vi "Viavi - Main.vi"(8 "error in (no error)":errorcluster {"code" format="Error %.0f"}, 10 "notifiers":T8, 11 "messageQueues":T9) -> (0 "error out":errorcluster {"code" format="Error %.0f"})   [LabVIEW 2017]
uses:
  Support/Configuration/Message Queues/messageQueues.ctl
  Support/Configuration/Message Queues/Message Cluster.ctl
  Support/Configuration/Notifiers/notifiers.ctl
  Controls/Viavi - Data.ctl
  Controls/Viavi - objectRefs.ctl
  Controls/Viavi - Instructions.ctl
  75e8a571-c33f-46d4-930b-ea0aecc2dba4.vi
  c46a4b58-3cb9-4cd0-a122-5f2cefd5d860.vi
  <vilib>/Utility/error.llb/Error Cluster From Error Code.vi
  <vilib>/ErrorRing/Error Ring.xnode
  Support/Configuration/User Events/User Event - Stop.lvlib
  Support/Configuration/Message Queues/Message Queue.lvlib
  <instrlib>/Viavi mORL-A1/Viavi mORL-A1.lvlib
  Support/Configuration/Notifiers/notifiers.lvlib
panel:
  in  "IL Warnings Enable":bool
  in  "IL Warning Values":cluster{"IL Min":dbl, "IL Max":dbl}={"IL Min"=0.0, "IL Max"=99.0}
  in  "Table Key":cluster{"Warning":bool, "Failure":bool}
  out "Data Error":string
  out "Method Selection":u16(ring) items=["Select Test Method", "---------------------", "Standard", "Substitution", "Cutback (placeholder)"]
  out "Testing Parameters":T1={"IL Param"={"Warning High"=inf, "Warning Low"=0.0, "Fail High"=0.0, "Fail Low"=-inf, "Display Precision"=2}, "RL Param"={"Warning High"=inf, "Warning Low"=35.0, "Fail High"=inf, "Fail Low"=0.0, "Display Precision"=1}, "RL2 Param"={"Warning High"=inf, "Warning Low"=35.0, "Fail High"=inf, "Fail Low"=-inf, "Display Precision"=1}, "Power Param"={"Warning High"=inf, "Warning Low"=-28.0, "Fail High"=inf, "Fail Low"=-inf, "Display Precision"=2}, "Length Param"={"Warning High"=inf, "Warning Low"=-inf, "Fail High"=inf, "Fail Low"=-inf, "Display Precision"=1}}
  out "pRatio Array":dbl[](array[numeric])
  out "Temp Ref Power Array":T2(array[cluster])
  out "Temp Power Array":T2(array[cluster])
  out "Temp RL2 Array":T2(array[cluster])
  out "Temp RL Array":T2(array[cluster])
  out "Temp IL Array":T2(array[cluster])
  out "Length Array":T2(array[cluster])
  out "Ref Length Array":T2(array[cluster])
  in  "Measure pRatio":bool
  in  "First Reference":bool=TRUE caption="Taken First Ref"
  out "Single Channel":bool
  out "Enable RL":bool
  out "Enable IL":bool
  out "Wavelength Enable":bool[](array[boolean])
  out "Channel Select":bool[](array[boolean])
  out "Has Switch":bool caption="Switch Installed"
  in  "Slot Number":i32=3
  out "Device ID":refnum<visa-resource-name>="GPIB0::17::INSTR"
  in  "displayTab":T3(tab)
  in  "Custom RL Cluster":T4 {"RL Method" items=["", "Input", "Output", "Between", "In + Out"]}
  in  "RL2 Standard":u16(ring) items=["Select RL2 Standard", "---------------------", "No Standard", "Custom Standard", "---------------------", "GR326-UPC-New ", "GR326-UPC-During/End", "GR326-APC-New ", "GR326-APC-During/End", "GR1435-Standard-New", "GR1435-Standard-During/End"]
  out "Both Image":picture
  out "Between Image":picture
  out "Output Image":picture
  out "Input Image":picture
  out "RL Presets":T5(radio)
  out "RL Configs":T6={"Measurement Mode"=FALSE, "Enable RL2"=FALSE, "RL1 Anchor Point"=enum."Left DUT Connection", "RL1 Measure Points"={-0.2500000000000009, 0.25}, "RL2 Anchor Point"=enum."Right DUT Connection", "RL2 Measure Points"={-0.2500000000000009, 0.25}} {"RL2 Measure Points" scale=-5.0..5.0 scale format="%#.2g"; "RL1 Measure Points" scale=-5.0..5.0 scale format="%#.2g"}
  out "Single Table":T7(array[cluster])
  out "Multi Ref/IL Table":T7(array[cluster])
  out "Multi RL Table":T7(array[cluster])
  out "Multi Ref/IL Columns":T2(array[cluster])=[{"String"="", "Warning"=FALSE, "Fail"=FALSE, "Numeric"=0.0}, {"String"="Ref: 1310", "Warning"=FALSE, "Fail"=FALSE, "Numeric"=0.0}, {"String"="Ref: 1490", "Warning"=FALSE, "Fail"=FALSE, "Numeric"=0.0}, {"String"="Ref: 1550", "Warning"=FALSE, "Fail"=FALSE, "Numeric"=0.0}, {"String"="Ref: 1625", "Warning"=FALSE, "Fail"=FALSE, "Numeric"=0.0}, {"String"="IL: 1310", "Warning"=FALSE, "Fail"=FALSE, "Numeric"=0.0}, {"String"="IL: 1490", "Warning"=FALSE, "Fail"=FALSE, "Numeric"=0.0}, {"String"="IL: 1550", "Warning"=FALSE, "Fail"=FALSE, "Numeric"=0.0}, {"String"="IL: 1625", "Warning"=FALSE, "Fail"=FALSE, "Numeric"=0.0}]
  out "Multi RL Columns":T2(array[cluster])=[{"String"="", "Warning"=FALSE, "Fail"=FALSE, "Numeric"=0.0}, {"String"="RL: 1310", "Warning"=FALSE, "Fail"=FALSE, "Numeric"=0.0}, {"String"="RL: 1490", "Warning"=FALSE, "Fail"=FALSE, "Numeric"=0.0}, {"String"="RL: 1550", "Warning"=FALSE, "Fail"=FALSE, "Numeric"=0.0}, {"String"="RL: 1625", "Warning"=FALSE, "Fail"=FALSE, "Numeric"=0.0}, {"String"="RL2: 1310", "Warning"=FALSE, "Fail"=FALSE, "Numeric"=0.0}, {"String"="RL2: 1490", "Warning"=FALSE, "Fail"=FALSE, "Numeric"=0.0}, {"String"="RL2: 1550", "Warning"=FALSE, "Fail"=FALSE, "Numeric"=0.0}, {"String"="RL2: 1625", "Warning"=FALSE, "Fail"=FALSE, "Numeric"=0.0}]
  in  "Instruction Button":bool
  out "Instruction Image":picture
  out "Instruction Text":string
  # "Custom RL\nOption"
  # "Select which point to measure"
  # "(if applicable)"
  # "Discrete"
  # "Integral"
  # "Left Point"
  # "Right Point"
  # "Left Point"
  # "Right Point"
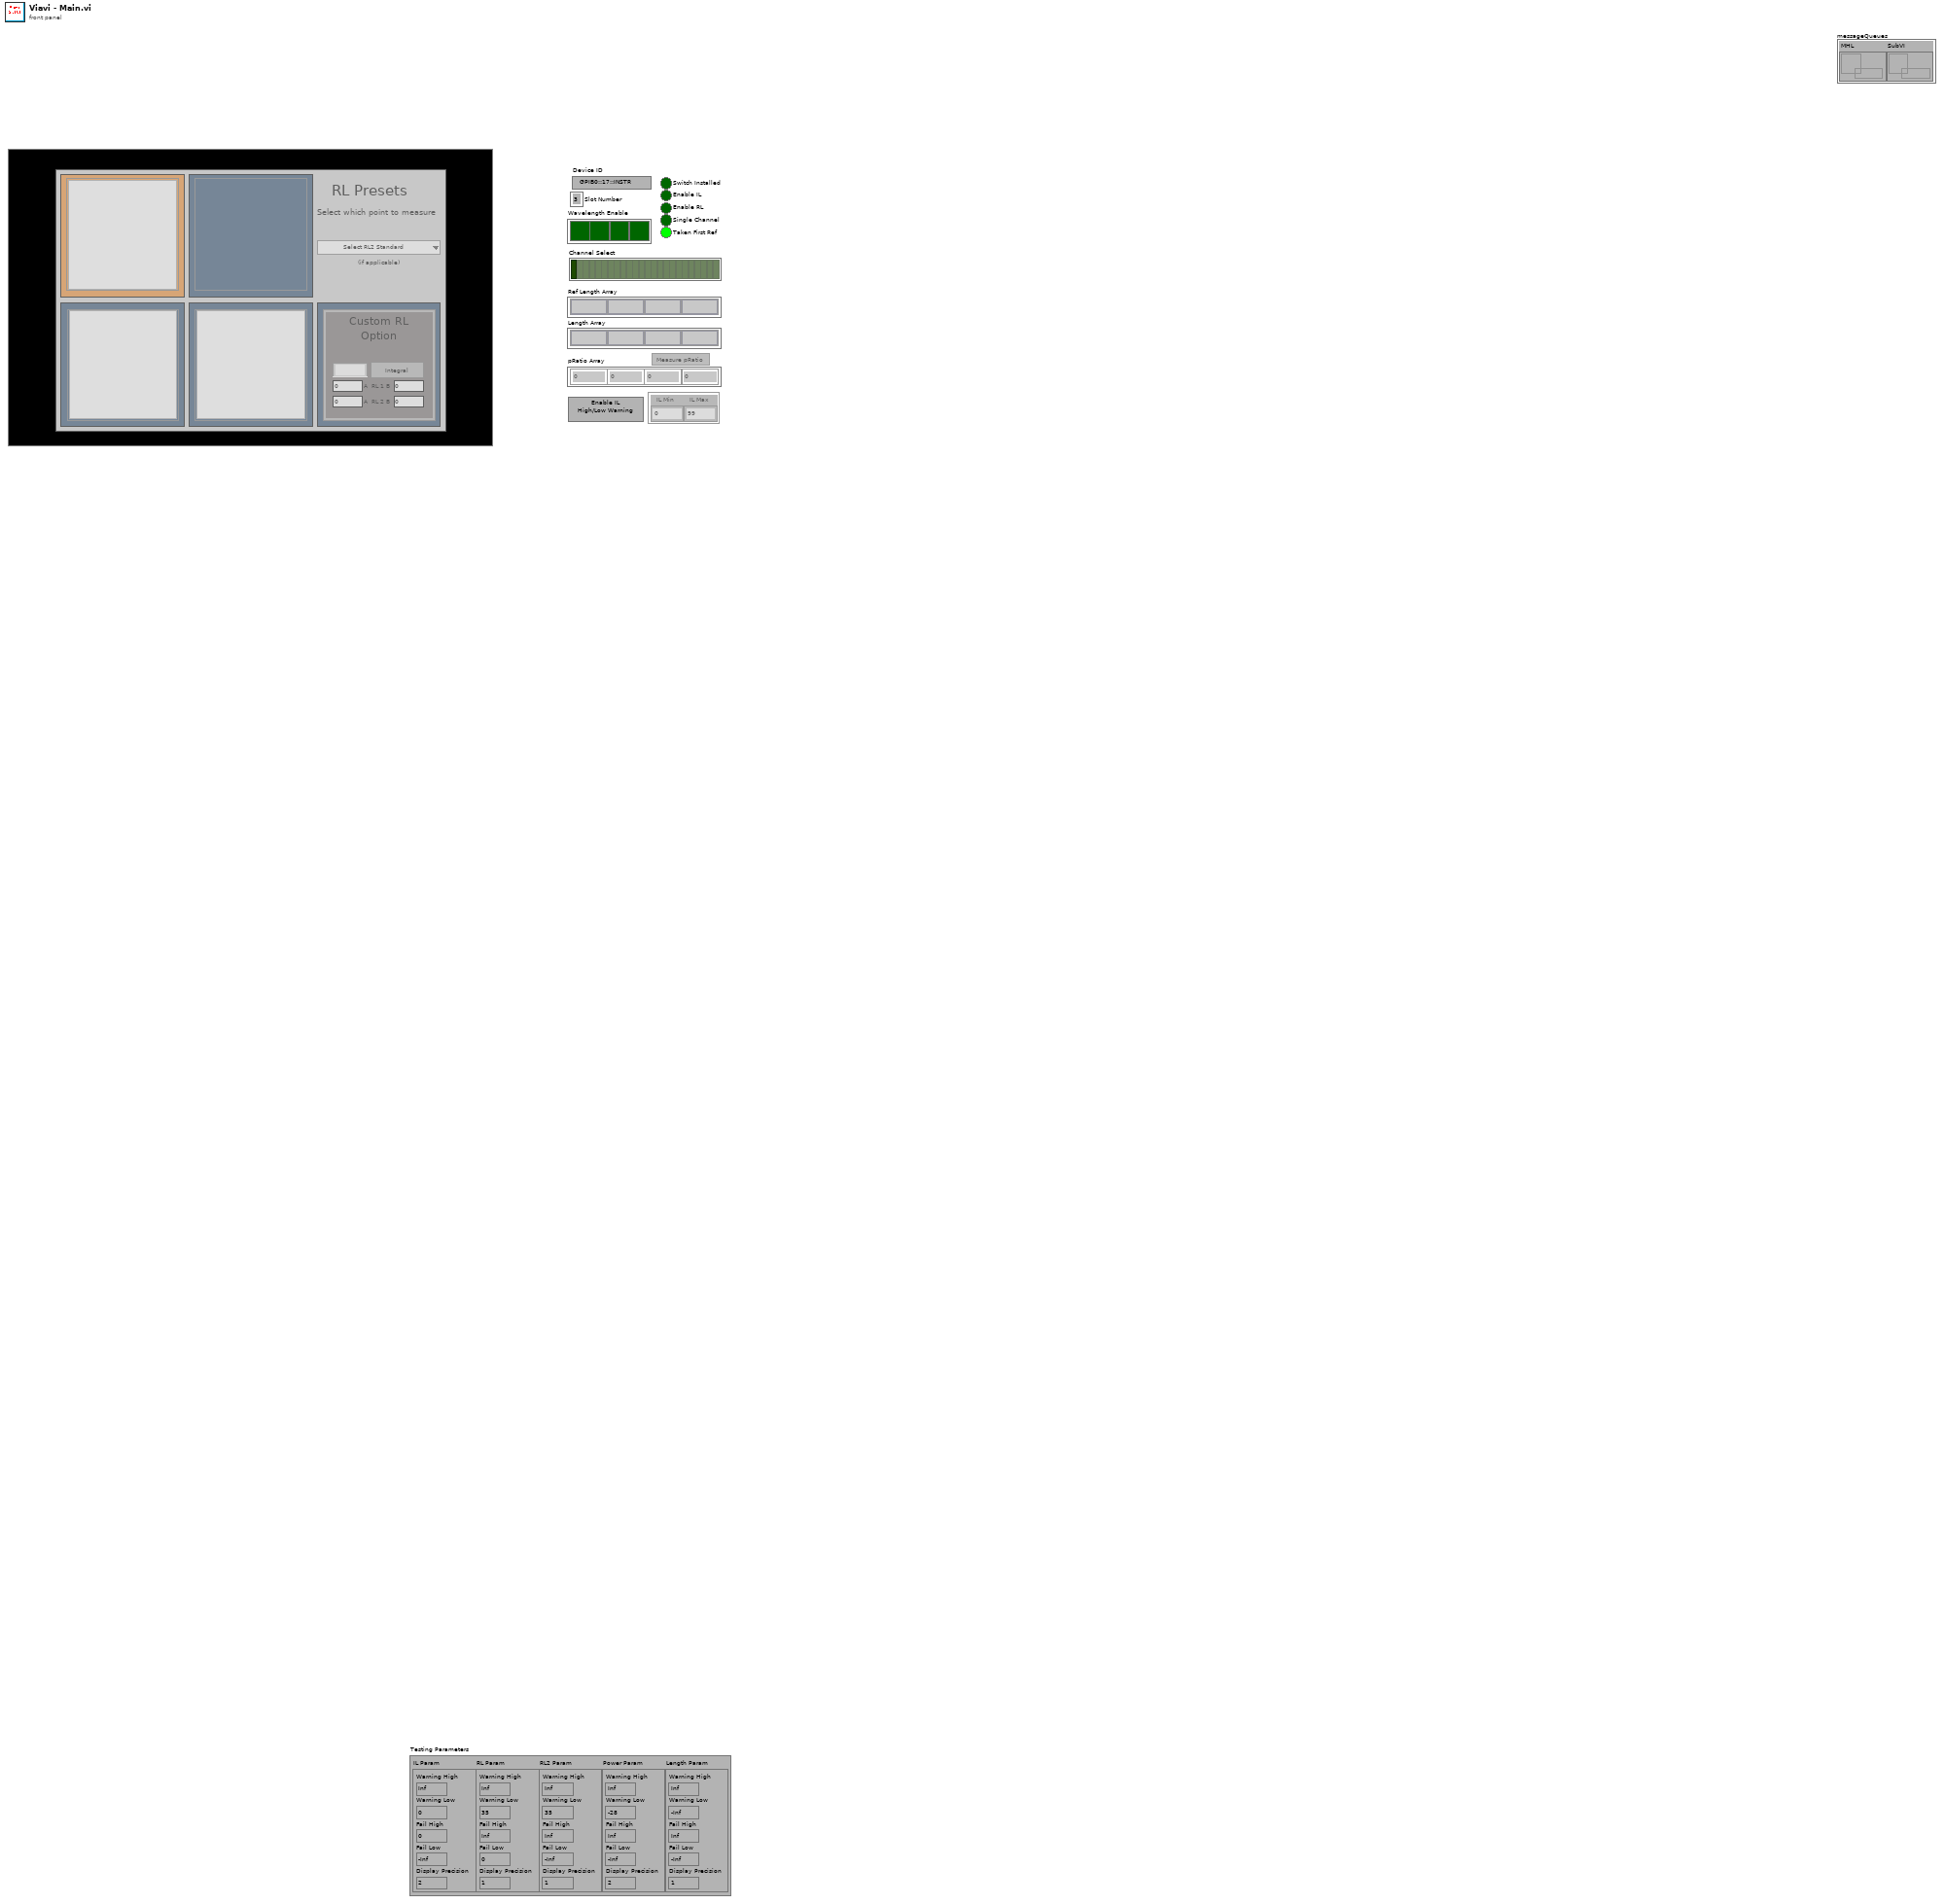
[diagram p1: front panel]
types:
  T1 = cluster{"IL Param":cluster{"Warning High":dbl, "Warning Low":dbl, "Fail High":dbl, "Fail Low":dbl, "Display Precision":i32}, "RL Param":cluster{"Warning High":dbl, "Warning Low":dbl, "Fail High":dbl, "Fail Low":dbl, "Display Precision":i32}, "RL2 Param":cluster{"Warning High":dbl, "Warning Low":dbl, "Fail High":dbl, "Fail Low":dbl, "Display Precision":i32}, "Power Param":cluster{"Warning High":dbl, "Warning Low":dbl, "Fail High":dbl, "Fail Low":dbl, "Display Precision":i32}, "Length Param":cluster{"Warning High":dbl, "Warning Low":dbl, "Fail High":dbl, "Fail Low":dbl, "Display Precision":i32}}
  T2 = cluster{"String":string, "Warning":bool, "Fail":bool, "Numeric":dbl}[]
  T3 = enum32{"RL Configs", "Data Table", "Instruction"}
  T4 = cluster{"Enable Integral":bool, "RL 1 A":dbl, "RL 1 B":dbl, "RL 2 A":dbl, "RL 2 B":dbl, "Enable RL2":bool, "RL Method":u16}
  T5 = enum32{"Left Anchor", "Right Anchor", "Center Anchor", "Left/Right Anchor", "Custom"}
  T6 = cluster{"Measurement Mode":bool, "Enable RL2":bool, "RL1 Anchor Point":enum32{"Left DUT Connection", "Right DUT Connection", "Center on DUT"}, "RL1 Measure Points":cluster{dbl, dbl}, "RL2 Anchor Point":enum32{"Left DUT Connection", "Right DUT Connection", "Center on DUT"}, "RL2 Measure Points":cluster{dbl, dbl}}
  T7 = cluster{"String":string, "Warning":bool, "Fail":bool, "Numeric":dbl}[][]
  T8 = typedef "notifiers.lvlib/notifiers.ctl" = cluster{"exitSubVI":refnum<notifier>}
  T9 = typedef "Message Queue.lvlib/messageQueues.ctl" = cluster{"MHL":refnum<queue>, "SubVI":refnum<queue>}
  T10 = typedef "Viavi - Data.ctl" = cluster{"Viavi - objectRefs":T11}
  T11 = typedef "Viavi - objectRefs.ctl" = cluster{"displayTab":refnum<vi>, "SubVI Pane":refnum<vi>, "instructStringRef":refnum<vi>, "instructImageRef":refnum<vi>, "instructButtonRef":refnum<vi>, "ResourceNameRef":refnum<vi>, "SlotNumberRef":refnum<vi>, "HasSwitchRef":refnum<vi>, "WavelengthRef":refnum<vi>, "SingleChannelRef":refnum<vi>, "IlEnableRef":refnum<vi>, "RlEnableRef":refnum<vi>, "RLConfigsRef":refnum<vi>, "RLPresetRef":refnum<vi>, "SingleTableRef":refnum<vi>, "MultiRef/ILTableRef":refnum<vi>, "MultiRLTableRef":refnum<vi>, "TempILRef":refnum<vi>, "TempRLRef":refnum<vi>, "TempRL2Ref":refnum<vi>, "TempRefPowRef":refnum<vi>, "TempPowRef":refnum<vi>, "RefLengthRef":refnum<vi>, "LengthArrayRef":refnum<vi>, "ChannelRef":refnum<vi>, "TestParamsRef":refnum<vi>, "MethodSelectRef":refnum<vi>, "DataErrorRef":refnum<vi>, "RL2StandardRef":refnum<vi>}
  T12 = typedef "User Event - Stop.lvlib/userEvents.ctl" = cluster{"stop":refnum<user-event>, "sendRefs":refnum<user-event>, "sendSubVIRefs":refnum<user-event>, "eventRegRef":refnum<event-registration>}
  T13 = cluster{"queueName":string, "queueMessage":string, "priority?":bool}[]
  T14 = enum8{"Enabled", "Disabled", "Disabled and Grayed Out"}
  T15 = cluster{"VISA resource name":refnum<visa-resource-name>, "HasSwitch":bool}
  T16 = cluster{"Wavelength Enable":bool[], "Channel Cluster":bool[], "Enable IL":bool, "Enable RL":bool, "Enable Switch":bool, "Method Selection":u16, "Value":cluster{"Standard Name":string, "Max IL to Pass (dB)":dbl, "Min RL to Pass (dB)":dbl}}
  T17 = typedef "Viavi - Instructions.ctl" = cluster{"Reference Instructions":cluster{"Instruction Text":string, "Instruction Image":picture, "Main Display Message":string}, "Reference (substitution) Instructions":cluster{"Instruction Text":string, "Instruction Image":picture, "Main Display Message":string}, "Reference (cutback) Instructions":cluster{"Instruction Text":string, "Instruction Image":picture, "Main Display Message":string}, "Measure Instructions":cluster{"Instruction Text":string, "Instruction Image":picture, "Main Display Message":string}, "Measure (Substitution) Instructions":cluster{"Instruction Text":string, "Instruction Image":picture, "Main Display Message":string}, "Measure (Cutback) Instructions":cluster{"Instruction Text":string, "Instruction Image":picture, "Main Display Message":string}, "Disconnect Int Sphere Instructions":cluster{"Instruction Text":string, "Instruction Image":picture, "Main Display Message":string}, "Connect Int Sphere Instructions":cluster{"Instruction Text":string, "Instruction Image 2":picture, "Main Display Message":string}, " Multichannel Reference Instructions":cluster{"Instruction Text":string, "Instruction Image":picture, "Main Display Message":string}, " Multichannel Reference (substitution) Instructions":cluster{"Instruction Text":string, "Instruction Image":picture, "Main Display Message":string}, " Multichannel Reference (cutback) Instructions":cluster{"Instruction Text":string, "Instruction Image":picture, "Main Display Message":string}, "Multichannel Measure Instructions":cluster{"Instruction Text":string, "Instruction Image":picture, "Main Display Message":string}, "Multichannel Measure (Substitution) Instructions":cluster{"Instruction Text":string, "Instruction Image":picture, "Main Display Message":string}, "Multichannel Measure (Cutback) Instructions":cluster{"Instruction Text":string, "Instruction Image":picture, "Main Display Message":string}}
  T18 = cluster{"Temp Ref Power Array":cluster{"String":string, "Warning":bool, "Fail":bool, "Numeric":dbl}[], "Temp IL Array":cluster{"String":string, "Warning":bool, "Fail":bool, "Numeric":dbl}[], "Temp RL Array":cluster{"String":string, "Warning":bool, "Fail":bool, "Numeric":dbl}[], "Temp RL2 Array":cluster{"String":string, "Warning":bool, "Fail":bool, "Numeric":dbl}[]}
  T19 = cluster{"IL Array":cluster{"Data Output":string, "Fail":bool}[], "RL Array":cluster{"Data Output":string, "Fail":bool}[], "Ref Power Array":string[], "Power Array":string[], "Optional Data Array":cluster{"Data Output":string, "Fail":bool}[], "Optional Param":string}
  T20 = cluster{"Standard Name":string, "Max IL to Pass (dB)":dbl, "Min RL to Pass (dB)":dbl}
  T21 = cluster{"String":string, "Warning":bool, "Fail":bool, "Numeric":dbl}
  T22 = cluster{"Measurement Mode":bool, "Enable RL2":bool, "RL1 Anchor Point":enum32{"Left DUT Connection", "Right DUT Connection", "Center on DUT"}, "RL1 Measure Points":cluster{"RL1 Left":dbl, "RL1 Right":dbl}, "RL2 Anchor Point":enum32{"Left DUT Connection", "Right DUT Connection", "Center on DUT"}, "RL2 Measure Points":cluster{"RL2 Left":dbl, "RL2 Right":dbl}}
  T23 = cluster{"Instruction Text":string, "Instruction Image":picture, "Main Display Message":string}[]
  T24 = cluster{"Instruction Text":string, "Instruction Image":picture, "Main Display Message":string}
  T25 = cluster{"Temp IL Array":cluster{"String":string, "Warning":bool, "Fail":bool, "Numeric":dbl}[], "Temp RL Array":cluster{"String":string, "Warning":bool, "Fail":bool, "Numeric":dbl}[], "Temp RL2 Array":cluster{"String":string, "Warning":bool, "Fail":bool, "Numeric":dbl}[], "Temp Power Array":cluster{"String":string, "Warning":bool, "Fail":bool, "Numeric":dbl}[], "Length Array":cluster{"String":string, "Warning":bool, "Fail":bool, "Numeric":dbl}[]}
  T26 = cluster{"Warning High":dbl, "Warning Low":dbl, "Fail High":dbl, "Fail Low":dbl, "Display Precision":i32}
  T27 = cluster{"Standard Name":string, "Max IL to Pass (dB)":dbl, "Min RL to Pass (dB)":dbl}[]
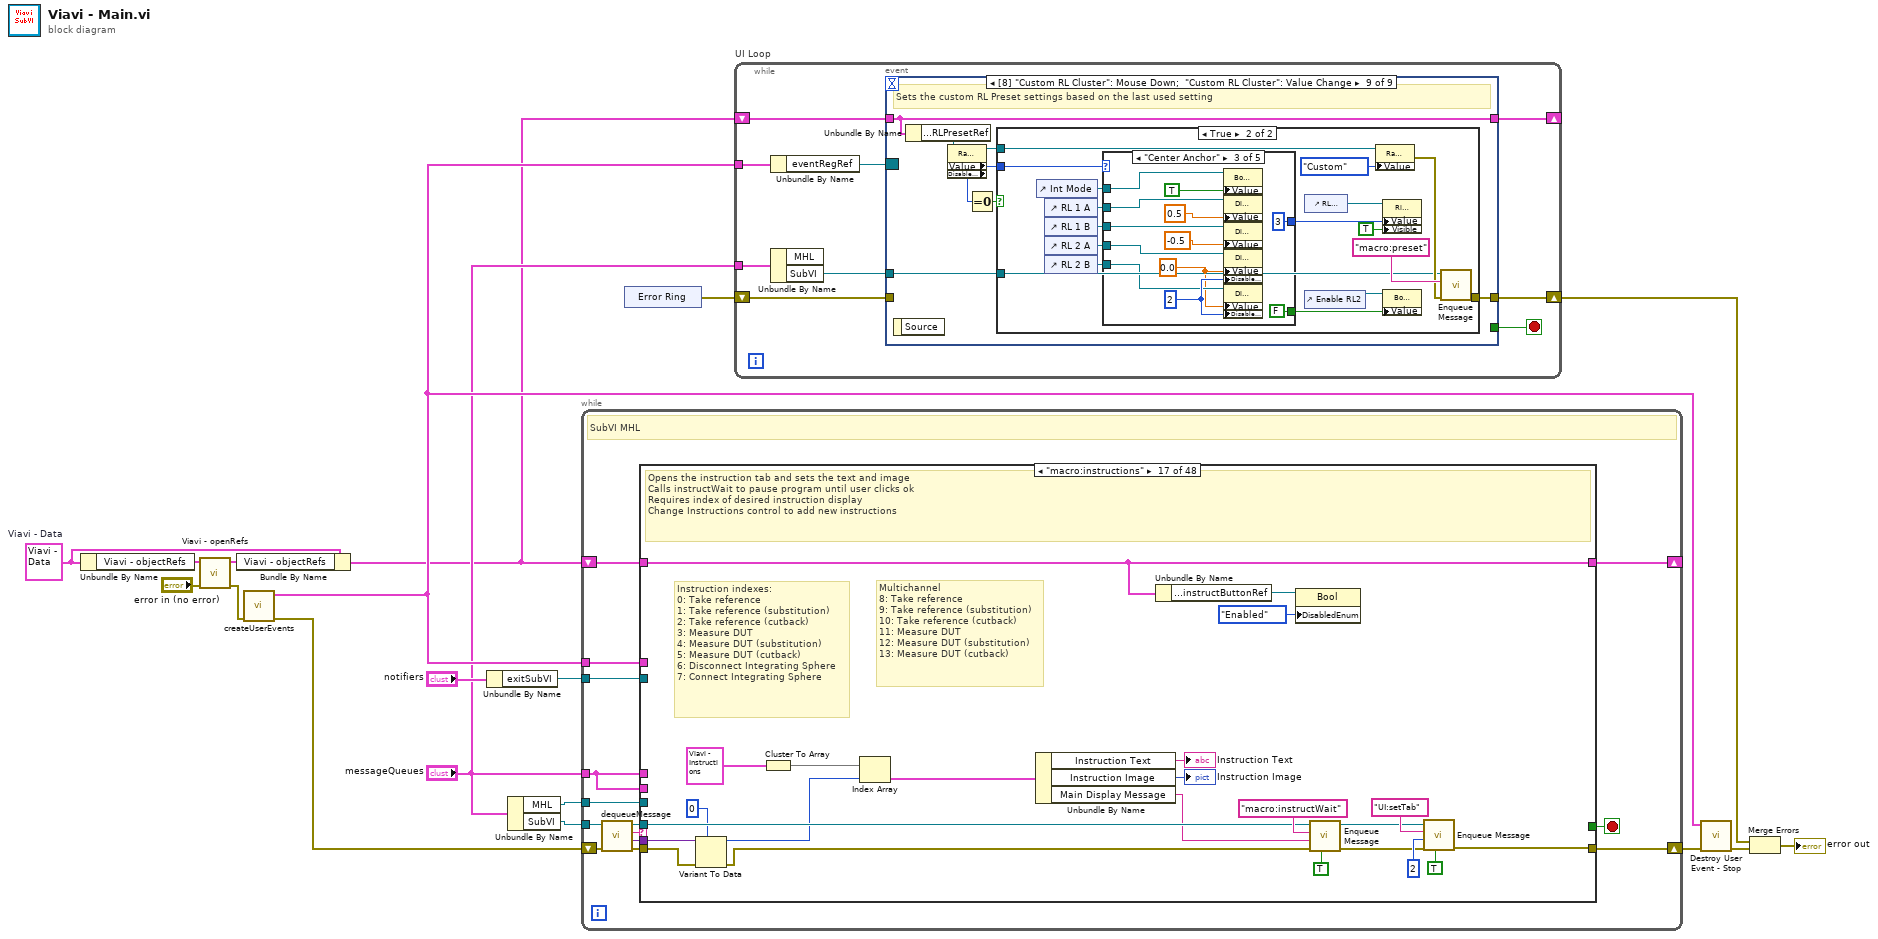
[diagram p0: block diagram]
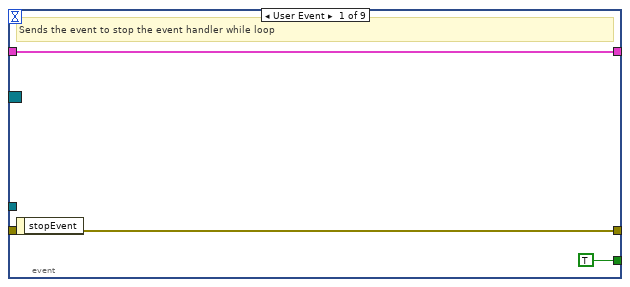
[diagram p2: hidden frame]
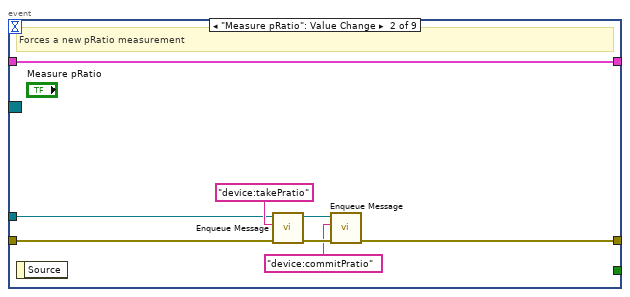
[diagram p3: hidden frame]
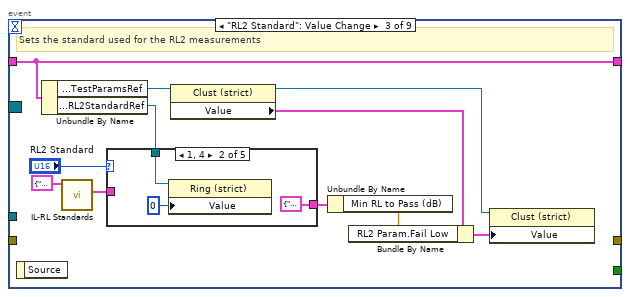
[diagram p4: hidden frame]
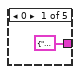
[diagram p5: hidden frame]
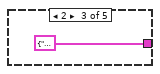
[diagram p6: hidden frame]
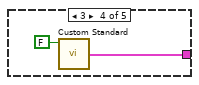
[diagram p7: hidden frame]
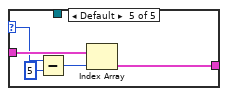
[diagram p8: hidden frame]
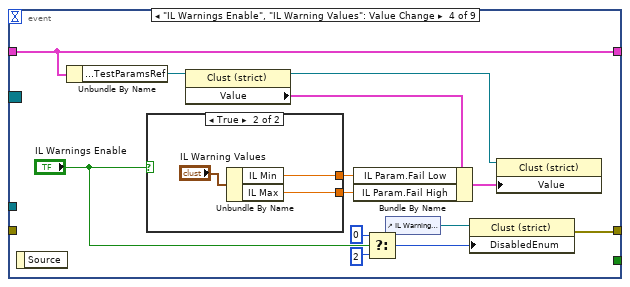
[diagram p9: hidden frame]
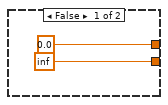
[diagram p10: hidden frame]
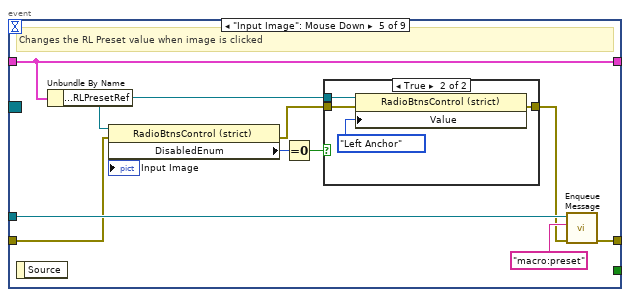
[diagram p11: hidden frame]
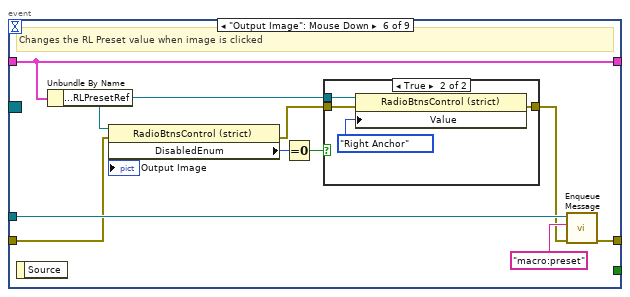
[diagram p13: hidden frame]
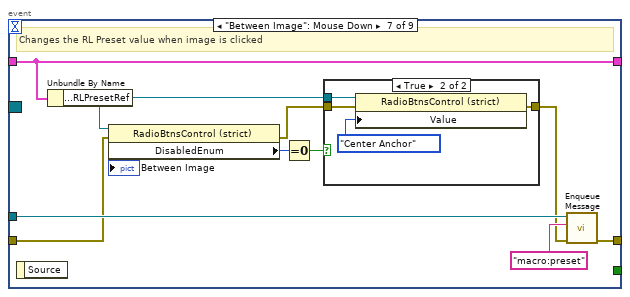
[diagram p15: hidden frame]
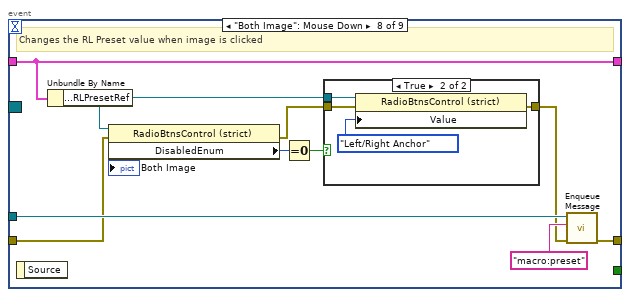
[diagram p17: hidden frame]
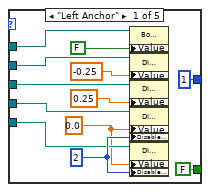
[diagram p20: hidden frame]
diagram:
  w5 = T10 {"Viavi - objectRefs"={"displayTab"=refnum, "SubVI Pane"=refnum, "instructStringRef"=refnum, "instructImageRef"=refnum, "instructButtonRef"=refnum, "ResourceNameRef"=refnum, "SlotNumberRef"=refnum, "HasSwitchRef"=refnum, "WavelengthRef"=refnum, "SingleChannelRef"=refnum, "IlEnableRef"=refnum, "RlEnableRef"=refnum, "RLConfigsRef"=refnum, "RLPresetRef"=refnum, "SingleTableRef"=refnum, "MultiRef/ILTableRef"=refnum, "MultiRLTableRef"=refnum, "TempILRef"=refnum, "TempRLRef"=refnum, "TempRL2Ref"=refnum, "TempRefPowRef"=refnum, "TempPowRef"=refnum, "RefLengthRef"=refnum, "LengthArrayRef"=refnum, "ChannelRef"=refnum, "TestParamsRef"=refnum, "MethodSelectRef"=refnum, "DataErrorRef"=refnum, "RL2StandardRef"=refnum}}  # Viavi - Data
  n1 = Unbundle By Name(w5) -> ("Viavi - objectRefs"=w6:T11)
  n2 = call "Viavi - openRefs.vi"("error in (no error)"="error in (no error)", "Viavi - strictRefs In"=w6) -> ("error out"=w2:errorcluster, "Viavi - strictRefs Out"=w4:T11)  [unwired: 6 in, 2 out]
  n3 = Bundle By Name(cluster=w5, "Viavi - objectRefs"=w4) -> (w1:T10)
  n4 = call "createUserEvents.vi"("error in (no error)"=w2) -> ("error out"=w14:errorcluster, "userEvents"=w8:T12)  [unwired: 9 in]
  n5 = Unbundle By Name("notifiers") -> ("exitSubVI"=w15:refnum<notifier>)
  n6 = Unbundle By Name("messageQueues") -> ("MHL"=w17:refnum<queue>, "SubVI"=w18:refnum<queue>)
  n7 = while {
    shift-right: [w19] -> w13
    shift-left: w14 -> [w32]
    tunnel: w18 -> [w27]
    tunnel: w17 -> [w30]
    shift-right: [w23] -> _
    shift-left: w1 -> [w24]
    tunnel: w15 -> [w22]
    tunnel: w8 -> [w21]
    tunnel: "messageQueues" -> [w20]
    stop <- w25 stop-if-true
    # "SubVI MHL"
    n8 = call "dequeueMessage.vi"("error in (no error)"=w32, "Message Queue"=w27) -> ("error out"=w31:errorcluster, "Message Data"=w28:variant, "Message"=w29:string, "dup Message Queue"=w26:refnum<queue>)  [unwired: 6 in]
    n9 = case "Rotation Cases" shown="\"macro:instructions\"" w29 {
      selector: w29 -> [_ _ _ _ _ _ _ _ _ _ _ _ _ _ _ _ _ _ _ _ w560 _ _ _ _ _ _ _ _ _ _ _ _ _ _ _ _ _ _ _ _ _ _ _ _ _ _ _]
      tunnel: w31 -> [w34 w42 w84 w109 w119 w136 w144 w170 w178 w214 w215 w217 w246 w275 w340 w410 w479 w483 w517 w558 _ w576 w595 w600 w604 w608 w617 w658 w693 w699 w729 w744 w777 w798 w807 w813 w820 w841 w857 w861 w870 w884 w891 w914 w919 w957 w976 w1012]
      tunnel: [w34 w44 w88 w111 w113 w138 w155 w169 w173 w201 w215 w224 w236 w280 w348 w404 w474 w486 w516 w558 w561 w571 w591 w600 w604 w608 w617 w643 w693 w698 w722 w736 w771 w792 w802 w813 w822 w838 w855 w860 w873 w879 w901 w910 w927 w942 w981 w1014] -> w19
      tunnel: w30 -> [_ _ _ w104 _ _ w150 _ _ _ _ _ _ _ _ _ _ w485 _ _ _ w572 _ _ _ _ _ w671 _ _ _ w743 w776 w797 _ _ _ _ _ _ _ _ w890 w913 _ _ _ _]
      tunnel: w28 -> [_ _ _ _ w121 _ w151 _ w177 w213 _ _ _ _ _ _ w478 w484 _ _ _ w575 _ _ _ _ _ _ _ _ w728 _ _ _ w806 _ w823 _ w856 _ w869 w883 _ _ _ w958 w980 w1017]
      tunnel: w26 -> [_ w43 w85 w108 _ w134 _ _ _ w204 _ w218 w241 w272 w341 w413 w470 w488 w515 _ _ _ w599 _ _ _ _ _ _ w697 _ w733 _ _ _ _ w824 _ w845 _ _ _ w894 _ w926 _ _ _]
      tunnel: [_ _ _ _ _ _ _ _ _ _ _ _ _ _ _ _ _ _ _ _ _ _ TRUE _ _ _ _ _ _ _ _ _ _ _ _ _ _ _ _ _ _ _ _ _ _ _ _ _] -> w25
      tunnel: w24 -> [w33 w38 w78 w112 w117 w140 w148 w171 w179 w191 w216 w225 w227 w285 w353 w409 w462 w482 w513 w559 w562 w580 w598 w601 w605 w614 w633 w668 w694 w710 w723 w740 w770 w791 w804 w812 w815 w842 w849 w864 w876 w887 w898 w916 w920 w956 w973 w1010]
      tunnel: [w33 w38 w78 w112 w117 w140 w148 w171 w179 w191 w216 w225 w227 w285 w353 w409 w462 w482 w513 w559 w562 w580 w598 w601 w605 w614 w633 w668 w694 w710 w723 w740 w770 w791 w804 w812 w815 w842 w849 w864 w876 w887 w898 w916 w920 w956 w973 w1010] -> w23
      tunnel: w22 -> [_ _ _ _ _ _ _ _ _ _ _ _ _ _ _ _ _ _ _ _ _ _ w597 _ _ _ _ _ _ _ _ _ _ _ _ _ _ _ _ _ _ _ _ _ _ _ _ _]
      tunnel: w21 -> [_ _ _ _ _ _ _ _ _ _ _ _ _ _ _ _ _ _ _ _ _ _ w590 _ _ _ _ _ _ _ _ _ _ _ _ _ _ _ _ _ _ _ _ _ _ _ _ _]
      tunnel: w20 -> [_ _ w87 w110 _ w132 w154 w168 _ _ _ w223 _ _ _ _ _ _ _ _ _ w570 _ _ _ _ _ _ _ _ _ _ _ _ _ _ _ _ _ _ _ _ _ _ _ _ _ _]
      tunnel: w20 -> [_ w45 _ _ _ _ _ _ _ _ _ _ _ _ _ _ _ _ _ _ _ _ _ _ _ _ _ _ _ _ _ _ _ _ _ _ _ _ _ _ _ _ _ _ _ _ _ _]
      frame "-------- Mandatory --------" {
        # "Template Separator\n(You can make a copy of, or modify, this frame)"
      }
      frame "macro:takeRef" {
        # "Runs an iteration of references and dataGets for each selected wavelength.\nIf first reference of SPN, check pRatio"
        n10 = Unbundle By Name(w38) -> ("Viavi - objectRefs.MethodSelectRef"=w41:refnum<vi>, "Viavi - objectRefs.SingleChannelRef"=w37:refnum<vi>)
        n11 = property class="Ring (strict)"(reference=w41) -> ("Value"=w40:u16)  [unwired: 1 in, 2 out]
        n12 = property class="Bool (strict)"(reference=w37) -> ("Value"=w36:bool)  [unwired: 1 in, 2 out]
        n13 = case shown="2, 3" w40 {
          tunnel: [_ w47 w51] -> w39
          tunnel: w36 -> [_ w48 w52]
          frame Default {
          }
          frame 2, 3 {
            # "Standard/Sub"
            n14 = Select(t=0, s=w48, f=8) -> (s? t:f=w47:i32)
          }
          frame 4 {
            # "Cutback"
            n15 = Select(t=2, s=w52, f=10) -> (s? t:f=w51:i32)
          }
        }
        n16 = case shown="False" "First Reference" {
          tunnel: w42 -> [w58 w67]
          tunnel: w43 -> [w56 w66]
          tunnel: [w57 w69] -> w44
          tunnel: w45 -> [_ w70]
          tunnel: T13 [{"queueName"="SubVI", "queueMessage"="data:cleanRefTemps", "priority?"=FALSE}, {"queueName"="SubVI", "queueMessage"="data:buildTable", "priority?"=FALSE}, {"queueName"="SubVI", "queueMessage"="macro:queueRef", "priority?"=FALSE}] ("queueMessages") -> [_ w68]
          tunnel: w39 -> [_ w59]
          frame True {
            n17 = call "Enqueue Message.vi"("error in (no error)"=w58, "Message"="macro:pRatio", "Message Queue"=w56) -> ("error out"=w57:errorcluster)  [unwired: 7 in, 1 out]
          }
          frame False {
            n18 = call "Enqueue Message.vi"("error in (no error)"=w67, "Message Data"=w59, "Message"="macro:instructions", "Message Queue"=w66) -> ("error out"=w62:errorcluster, "dup Message Queue"=w60:refnum<queue>)  [unwired: 6 in]
            n19 = call "Enqueue Message.vi"("error in (no error)"=w62, "Message Data"=1, "Message"="UI:setTab", "Message Queue"=w60) -> ("error out"=w61:errorcluster)  [unwired: 6 in, 1 out]
            n20 = call "sendMultipleMessages.vi"("error in (no error)"=w61, "queueMessages"=w68, "messageQueues"=w70) -> ("error out"=w69:errorcluster)  [unwired: 8 in]
          }
        }
      }
      frame "macro:takeMeas" {
        # "Runs an iteration of measurements and dataGets for each selected wavelength."
        n21 = Unbundle By Name(w78) -> ("Viavi - objectRefs.DataErrorRef"=w77:refnum<vi>, "Viavi - objectRefs.MethodSelectRef"=w72:refnum<vi>, "Viavi - objectRefs.SingleChannelRef"=w73:refnum<vi>)
        n22 = property class="Str"(reference=w77, "Value"="") -> ()  [unwired: 1 in, 2 out]
        n23 = property class="Ring (strict)"(reference=w72) -> ("Value"=w75:u16)  [unwired: 1 in, 2 out]
        n24 = property class="Bool (strict)"(reference=w73) -> ("Value"=w74:bool)  [unwired: 1 in, 2 out]
        n25 = case shown="2" w75 {
          tunnel: [_ w90 w94 w98] -> w71
          tunnel: w74 -> [_ w91 w95 w99]
          frame Default {
          }
          frame 2 {
            # "Standard"
            n26 = Select(t=3, s=w91, f=11) -> (s? t:f=w90:i32)
          }
          frame 3 {
            # "Substitution"
            n27 = Select(t=4, s=w95, f=12) -> (s? t:f=w94:i32)
          }
          frame 4 {
            # "Cutback"
            n28 = Select(t=5, s=w99, f=13) -> (s? t:f=w98:i32)
          }
        }
        n29 = call "Enqueue Message.vi"("error in (no error)"=w84, "Message Data"=w71, "Message"="macro:instructions", "Message Queue"=w85) -> ("error out"=w82:errorcluster, "dup Message Queue"=w83:refnum<queue>)  [unwired: 6 in]
        n30 = call "Enqueue Message.vi"("error in (no error)"=w82, "Message Data"=1, "Message"="UI:setTab", "Message Queue"=w83) -> ("error out"=w79:errorcluster)  [unwired: 6 in, 1 out]
        n31 = call "sendMultipleMessages.vi"("error in (no error)"=w79, "queueMessages"=T13 [{"queueName"="SubVI", "queueMessage"="data:cleanMeasTemps", "priority?"=FALSE}, {"queueName"="SubVI", "queueMessage"="data:buildTable", "priority?"=FALSE}, {"queueName"="SubVI", "queueMessage"="macro:queueMeas", "priority?"=FALSE}], "messageQueues"=w87) -> ("error out"=w88:errorcluster)  [unwired: 8 in]
      }
      frame "macro:abort" {
        # "Clears all messages from the SubVI queue\nAborts the devices current measurement and removes last temp data"
        n32 = Flush Queue(queue=w108, error in (no error)=w109) -> (error out=w106:errorcluster)  [unwired: 2 out]
        n33 = call "Enqueue Message.vi"("error in (no error)"=w106, "Message Data"="Device processes aborted" ("Message"), "Message"="UI:updateDisplay", "Message Queue"=w104) -> ("error out"=w105:errorcluster)  [unwired: 6 in, 1 out]
        n34 = call "sendMultipleMessages.vi"("error in (no error)"=w105, "queueMessages"=T13 [{"queueName"="SubVI", "queueMessage"="device:abort", "priority?"=TRUE}], "messageQueues"=w110) -> ("error out"=w111:errorcluster)  [unwired: 8 in]
      }
      frame "macro:engMode" {
        # "Enables engineering mode functions"
        n35 = Variant To Data(error in=w119, type=TRUE, Variant=w121) -> (data=w118:bool, error out=w114:errorcluster)
        n36 = Unbundle By Name(w117) -> ("Viavi - objectRefs.displayTab"=w116:refnum<vi>)
        n37 = control-ref of="Measure pRatio"() -> (w115:refnum<vi>)
        n38 = case shown="False" w118 {
          selector: w118 -> [w124 w129]
          tunnel: w116 -> [w126 w131]
          tunnel: w115 -> [w125 w130]
          tunnel: w114 -> [w122 w127]
          tunnel: [w122 w127] -> w113
          frame True {
            n39 = property class="TabCtl (strict)"(reference=w126, "Tabs Visible?"=w124) -> ()  [unwired: 1 in, 2 out]
            n40 = property class="Bool"(reference=w125, "DisabledEnum"=T14."Enabled" ("Disabled")) -> ()  [unwired: 1 in, 2 out]
          }
          frame False {
            n41 = property class="TabCtl (strict)"(reference=w131, "Tabs Visible?"=w129) -> ()  [unwired: 1 in, 2 out]
            n42 = property class="Bool"(reference=w130, "DisabledEnum"=T14."Disabled and Grayed Out" ("Disabled")) -> ()  [unwired: 1 in, 2 out]
          }
        }
      }
      frame "macro:newTest" {
        # "Reinitializes values to default to begin testing for a new Test"
        n43 = call "Enqueue Message.vi"("error in (no error)"=w136, "Message Data"=0, "Message"="UI:setTab", "Message Queue"=w134) -> ("error out"=w135:errorcluster)  [unwired: 6 in, 1 out]
        n44 = call "sendMultipleMessages.vi"("error in (no error)"=w135, "queueMessages"=T13 [{"queueName"="SubVI", "queueMessage"="data:cleanRefTemps", "priority?"=FALSE}, {"queueName"="SubVI", "queueMessage"="data:cleanMeasTemps", "priority?"=FALSE}, {"queueName"="SubVI", "queueMessage"="UI:initConfig", "priority?"=FALSE}], "messageQueues"=w132) -> ("error out"=w138:errorcluster)  [unwired: 8 in]
      }
      frame "macro:save" {
        # "Optional Save data used\nif RL2 is enabled"
        # "Trigger sending of current data to main.\nRuns build save if passed boolean indicates no current save file\nPasses 2d string array for RL2 save column names if RL2 is enabled\nRequires boolean indicating whether there is an active save file"
        n45 = Variant To Data(error in=w144, type=TRUE, Variant=w151) -> (data=w149:bool, error out=w145:errorcluster)
        n46 = Unbundle By Name(w148) -> ("Viavi - objectRefs.RLConfigsRef"=w147:refnum<vi>)
        n47 = property class="Clust (strict)"(reference=w147, error in=w144) -> ("Value"=w146:T22)  [unwired: 2 out]
        n48 = Unbundle By Name(w146) -> ("Enable RL2"=w143:bool)
        n49 = case shown="False" w143 {
          tunnel: [string[][] [] w157] -> w142
          tunnel: string[][] [["RL-2 (db)", "RL-2 (db)", "RL-2 (db)", "RL-2 (db)", "RL-2 Pass/Fail", "RL-2 Pass/Fail", "RL-2 Pass/Fail", "RL-2 Pass/Fail", "RL2 Pass"], ["1310nm", "1490nm", "1550nm", "1625nm", "1310nm", "1490nm", "1550nm", "1625nm", "Parameter"]] -> [_ w157]
          frame False {
          }
          frame True {
          }
        }
        n50 = case shown="False" w149 {
          tunnel: [w161 w166] -> w155
          tunnel: w154 -> [_ w165]
          tunnel: T13 [{"queueName"="SubVI", "queueMessage"="data:sendSaveData", "priority?"=FALSE}, {"queueName"="SubVI", "queueMessage"="data:cleanMeasTemps", "priority?"=FALSE}] ("queueMessages") -> [_ w164]
          tunnel: w145 -> [w162 w163]
          tunnel: w150 -> [w160 _]
          tunnel: w142 -> [w158 _]
          frame True {
            # "Build save headers"
            n51 = call "Enqueue Message.vi"("error in (no error)"=w162, "Message Data"=w158, "Message"="data:buildSave", "Message Queue"=w160) -> ("error out"=w161:errorcluster)  [unwired: 6 in, 1 out]
          }
          frame False {
            n52 = call "sendMultipleMessages.vi"("error in (no error)"=w163, "queueMessages"=w164, "messageQueues"=w165) -> ("error out"=w166:errorcluster)  [unwired: 8 in]
          }
        }
      }
      frame "macro:exit" {
        # "Shutdown procedure."
        n53 = call "sendMultipleMessages.vi"("error in (no error)"=w170, "queueMessages"=T13 [{"queueName"="SubVI", "queueMessage"="core:exit", "priority?"=FALSE}], "messageQueues"=w168) -> ("error out"=w169:errorcluster)  [unwired: 8 in]
      }
      frame "data:getInit" {
        # "Receives init variables from Main VI"
        n54 = Variant To Data(error in=w178, type=T15 {"VISA resource name"="", "HasSwitch"=FALSE} ("output cluster"), Variant=w177) -> (data=w175:T15, error out=w173:errorcluster)
        n55 = Unbundle By Name(w175) -> ("VISA resource name"=→"Device ID":refnum<visa-resource-name>, "HasSwitch"=→"Has Switch":bool)
      }
      frame "data:getConfig" {
        # "Receives config variables from Main VI\nHides data tables depending on single or multichannel\nDisables RL mode on device and UI if RL is disabled"
        n56 = Variant To Data(error in=w214, type=T16 {"Wavelength Enable"=[], "Channel Cluster"=[], "Enable IL"=FALSE, "Enable RL"=FALSE, "Enable Switch"=FALSE, "Method Selection"=0, "Value"={"Standard Name"="", "Max IL to Pass (dB)"=0.0, "Min RL to Pass (dB)"=0.0}} ("output cluster"), Variant=w213) -> (data=w212:T16, error out=w202:errorcluster)
        n57 = Unbundle By Name(w212) -> ("Wavelength Enable"=→"Wavelength Enable":bool[], "Channel Cluster"=→"Channel Select":bool[], "Enable IL"=→"Enable IL":bool, "Enable RL"=w185:bool, "Enable Switch"=w205:bool, "Method Selection"=→"Method Selection":u16, "Value"=w196:T20)
        "Enable RL" <- w185
        n58 = Unbundle By Name(w191) -> ("Viavi - objectRefs.SingleTableRef"=w208:refnum<vi>, "Viavi - objectRefs.MultiRef/ILTableRef"=w200:refnum<vi>, "Viavi - objectRefs.MultiRLTableRef"=w199:refnum<vi>)
        n59 = Not(x=w205) -> (.not. x?=w180:bool)
        "Single Channel" <- w180
        n60 = Not(x=w180) -> (.not. x?=w206:bool)
        n61 = Not(x=w180) -> (.not. x?=w207:bool)
        n62 = property class="Arr (strict)"(reference=w208, "Visible"=w180) -> ()  [unwired: 1 in, 2 out]
        n63 = property class="Arr (strict)"(reference=w200, "Visible"=w206) -> ()  [unwired: 1 in, 2 out]
        n64 = property class="Arr (strict)"(reference=w199, "Visible"=w207) -> ()  [unwired: 1 in, 2 out]
        n65 = control-ref of="Multi RL Columns"() -> (w184:refnum<vi>)
        n66 = control-ref of="Multi Ref/IL Columns"() -> (w183:refnum<vi>)
        n67 = call "Enqueue Message.vi"("error in (no error)"=w202, "Message Data"=w185, "Message"="device:ILOnly", "Message Queue"=w204) -> ("error out"=w201:errorcluster, "dup Message Queue"=w186:refnum<queue>)  [unwired: 6 in]
        n68 = call "Enqueue Message.vi"("Message Data"=w185, "Message"="UI:disableRL", "Message Queue"=w186) -> ()  [unwired: 7 in, 2 out]
        n69 = Select(t=-28.0, s=w180, f=-55.0) -> (s? t:f=w190:dbl)
        n70 = Not(x=w180) -> (.not. x?=w182:bool)
        n71 = Not(x=w180) -> (.not. x?=w181:bool)
        n72 = Unbundle By Name(w196) -> ("Max IL to Pass (dB)"=w195:dbl, "Min RL to Pass (dB)"=w194:dbl)
        n73 = property class="Arr (strict)"(reference=w184, "Visible"=w182) -> ()  [unwired: 1 in, 2 out]
        n74 = property class="Arr (strict)"(reference=w183, "Visible"=w181) -> ()  [unwired: 1 in, 2 out]
        n75 = Bundle By Name(cluster=T1 {"IL Param"={"Warning High"=inf, "Warning Low"=0.0, "Fail High"=inf, "Fail Low"=-inf, "Display Precision"=2}, "RL Param"={"Warning High"=inf, "Warning Low"=35.0, "Fail High"=inf, "Fail Low"=-inf, "Display Precision"=1}, "RL2 Param"={"Warning High"=inf, "Warning Low"=35.0, "Fail High"=inf, "Fail Low"=-inf, "Display Precision"=1}, "Power Param"={"Warning High"=inf, "Warning Low"=-inf, "Fail High"=inf, "Fail Low"=-inf, "Display Precision"=2}, "Length Param"={"Warning High"=inf, "Warning Low"=-inf, "Fail High"=inf, "Fail Low"=-inf, "Display Precision"=1}} ("Warning/Error Params"), "Power Param.Warning Low"=w190, "IL Param.Fail High"=w195, "RL Param.Fail Low"=w194) -> (→"Testing Parameters":T1)
      }
      frame "---------- Macro ----------" {
        # "Template Separator\n(You can make a copy of, or modify, this frame)"
      }
      frame "macro:init" {
        # "Startup procedure."
        n76 = call "Enqueue Message.vi"("error in (no error)"=w217, "Message Data"=FALSE, "Message"="macro:engMode", "Message Queue"=w218) -> ("error out"=w219:errorcluster)  [unwired: 6 in, 1 out]
        n77 = call "sendMultipleMessages.vi"("error in (no error)"=w219, "queueMessages"=T13 [{"queueName"="SubVI", "queueMessage"="device:init", "priority?"=FALSE}, {"queueName"="SubVI", "queueMessage"="macro:preset", "priority?"=FALSE}], "messageQueues"=w223) -> ("error out"=w224:errorcluster)  [unwired: 8 in]
      }
      frame "macro:pRatio" {
        # "Gets the current pRatio values\nAverages pRatio values and determines whether a new pRatio reference is needed\nand whether the integrating sphere needs to be connected or removed"
        n78 = Unbundle By Name(w227) -> ("Viavi - objectRefs.SingleChannelRef"=w247:refnum<vi>, "Viavi - objectRefs.ResourceNameRef"=w229:refnum<vi>, "Viavi - objectRefs.SlotNumberRef"=w228:refnum<vi>)
        n79 = property class="Bool (strict)"(reference=w247, error in=w246) -> ("Value"=w239:bool)  [unwired: 2 out]
        n80 = property class="VISAName"(reference=w229, error in=w246) -> ("Value"=w248:refnum<visa-resource-name>)  [unwired: 2 out]
        n81 = property class="DigNum (strict)"(reference=w228, error in=w246) -> ("Value"=w249:i32)  [unwired: 2 out]
        n82 = call <instrlib>:"Get PRatio.vi"("error in (no error)"=w246, "MAP-200 Slot Number"=w249, "VISA resource name"=w248) -> ("error out"=w242:errorcluster, "Initial Ratio"=w230:dbl[])  [unwired: 4 in, 3 out]
        "pRatio Array" <- w230
        n83 = Add Array Elements(numeric array=w230) -> (sum=w245:dbl)
        n84 = Divide(x=w245, y=4.0) -> (x/y=w233:dbl)
        n85 = Unbundle By Name(w227) -> ("Viavi - objectRefs.instructButtonRef"=w226:refnum<vi>)
        n86 = Greater Than 0?(x=w233) -> (x > 0?=w243:bool)
        n87 = Not Equal?(x=w239, y=w243) -> (x != y?=w240:bool)
        n88 = Select(t=6, s=w239, f=7) -> (s? t:f=w238:i32)
        n89 = case shown="False" w240 {
          tunnel: w242 -> [w254 w270]
          tunnel: w241 -> [w253 w268]
          tunnel: w238 -> [_ w267]
          tunnel: [w256 w261] -> w237
          tunnel: [w253 w260] -> w235
          tunnel: w226 -> [w250 w258]
          frame False {
            n90 = control-ref of="First Reference"() -> (w255:refnum<vi>)
            n91 = property class="Bool (strict)"(reference=w255, error in=w254, "Value"=FALSE) -> (error out=w256:errorcluster)  [unwired: 1 out]
            n92 = property class="Bool"(reference=w250, "DisabledEnum"=T14."Enabled" ("Disabled")) -> ()  [unwired: 1 in, 2 out]
          }
          frame True {
            n93 = call "Enqueue Message.vi"("error in (no error)"=w270, "Message Data"=w267, "Message"="macro:instructions", "Message Queue"=w268) -> ("error out"=w266:errorcluster, "dup Message Queue"=w265:refnum<queue>)  [unwired: 6 in]
            n94 = call "Enqueue Message.vi"("error in (no error)"=w266, "Message"="device:takePratio", "Message Queue"=w265) -> ("error out"=w262:errorcluster, "dup Message Queue"=w263:refnum<queue>)  [unwired: 7 in]
            n95 = property class="Bool"(reference=w258, "DisabledEnum"=T14."Disabled and Grayed Out" ("Disabled")) -> ()  [unwired: 1 in, 2 out]
            n96 = call "Enqueue Message.vi"("error in (no error)"=w262, "Message"="device:commitPratio", "Message Queue"=w263) -> ("error out"=w261:errorcluster, "dup Message Queue"=w260:refnum<queue>)  [unwired: 7 in]
          }
        }
        n97 = call "Enqueue Message.vi"("error in (no error)"=w237, "Message"="macro:takeRef", "Message Queue"=w235) -> ("error out"=w236:errorcluster)  [unwired: 7 in, 1 out]
      }
      frame "macro:queueRef" {
        # "Queues the messages necessary for referencing and dataGets for each selected wavelength per channel"
        n98 = Unbundle By Name(w285) -> ("Viavi - objectRefs.ChannelRef"=w278:refnum<vi>, "Viavi - objectRefs.WavelengthRef"=w277:refnum<vi>)
        n99 = call "Enqueue Message.vi"("error in (no error)"=w275, "Message Data"=FALSE, "Message"="device:multiJumper", "Message Queue"=w272) -> ("error out"=w274:errorcluster, "dup Message Queue"=w273:refnum<queue>)  [unwired: 6 in]
        n100 = property class="Arr (strict)"(reference=w277) -> ("Value"=w286:bool[])  [unwired: 1 in, 2 out]
        n101 = property class="Arr (strict)"(reference=w278) -> ("Value"=w284:bool[])  [unwired: 1 in, 2 out]
        n102 = Array Size(array=w284) -> (size(s)=w283:i32)
        n103 = for "Channel Loop" {
          N: w283 -> [_]
          tunnel: i32[] [1310, 1490, 1550, 1625] -> [w296]
          tunnel: w273 -> [w293]
          tunnel: w286 -> [w291]
          shift-right: [w295] -> w281
          shift-left: w274 -> [w292]
          tunnel: w284 -> [w290] mode=indexing
          tunnel: [w288] -> w279
          i -> [w294]
          n104 = Increment(x=w294) -> (x+1=w289:i32)
          n105 = case shown="True" w290 {
            tunnel: w296 -> [_ w309]
            tunnel: [w298 w308] -> w295
            tunnel: w293 -> [w297 w307]
            tunnel: w292 -> [w298 w305]
            tunnel: w291 -> [_ w302]
            tunnel: w289 -> [_ w299]
            tunnel: [w297 w300] -> w288
            frame False {
            }
            frame True {
              n106 = Array Size(array=w302) -> (size(s)=w301:i32)
              n107 = call "Enqueue Message.vi"("error in (no error)"=w305, "Message Data"=w299, "Message"="device:switch", "Message Queue"=w307) -> ("error out"=w304:errorcluster, "dup Message Queue"=w306:refnum<queue>)  [unwired: 6 in]
              n108 = for "Wavelength Loop" {
                N: w301 -> [_]
                tunnel: w302 -> [w322] mode=indexing
                tunnel: w309 -> [w321] mode=indexing
                tunnel: w306 -> [w320]
                shift-right: [w313] -> w308
                shift-left: w304 -> [w319]
                tunnel: [w314] -> w300
                n109 = case shown="True" w322 {
                  selector: w322 -> [w325 w327]
                  tunnel: w321 -> [_ w330]
                  tunnel: w320 -> [w324 w331]
                  tunnel: [w323 w329] -> w318
                  tunnel: [w324 w328] -> w317
                  tunnel: [w325 w327] -> w316
                  tunnel: w319 -> [w323 w326]
                  frame False {
                  }
                  frame True {
                    n110 = call "Enqueue Message.vi"("error in (no error)"=w326, "Message Data"=w330, "Message"="device:reference", "Message Queue"=w331) -> ("error out"=w329:errorcluster, "dup Message Queue"=w328:refnum<queue>)  [unwired: 6 in]
                  }
                }
                n111 = call "Enqueue Message.vi"("error in (no error)"=w318, "Message Data"=w316, "Message"="device:getRefData", "Message Queue"=w317) -> ("error out"=w310:errorcluster, "dup Message Queue"=w311:refnum<queue>)  [unwired: 6 in]
                n112 = call "Enqueue Message.vi"("error in (no error)"=w310, "Message"="data:buildTable", "Message Queue"=w311) -> ("error out"=w313:errorcluster, "dup Message Queue"=w314:refnum<queue>)  [unwired: 7 in]
              }
            }
          }
        }
        n113 = call "Enqueue Message.vi"("error in (no error)"=w281, "Message"="UI:endRef", "Message Queue"=w279) -> ("error out"=w280:errorcluster)  [unwired: 7 in, 1 out]
      }
      frame "macro:queueSubstRef" {
        # "Queues the messages necessary for referencing the input cable and dataGets for each selected wavelength per channel"
        n114 = Unbundle By Name(w353) -> ("Viavi - objectRefs.ChannelRef"=w346:refnum<vi>, "Viavi - objectRefs.WavelengthRef"=w345:refnum<vi>)
        n115 = call "Enqueue Message.vi"("error in (no error)"=w340, "Message"="data:cleanRefTemps", "Message Queue"=w341) -> ("error out"=w339:errorcluster, "dup Message Queue"=w338:refnum<queue>)  [unwired: 7 in]
        n116 = property class="Arr (strict)"(reference=w345) -> ("Value"=w354:bool[])  [unwired: 1 in, 2 out]
        n117 = property class="Arr (strict)"(reference=w346) -> ("Value"=w352:bool[])  [unwired: 1 in, 2 out]
        n118 = call "Enqueue Message.vi"("error in (no error)"=w339, "Message Data"=TRUE, "Message"="device:multiJumper", "Message Queue"=w338) -> ("error out"=w334:errorcluster, "dup Message Queue"=w335:refnum<queue>)  [unwired: 6 in]
        n119 = call "Enqueue Message.vi"("error in (no error)"=w334, "Message"="data:buildTable", "Message Queue"=w335) -> ("error out"=w337:errorcluster, "dup Message Queue"=w336:refnum<queue>)  [unwired: 7 in]
        n120 = Array Size(array=w352) -> (size(s)=w351:i32)
        n121 = for "Channel Loop" {
          N: w351 -> [_]
          tunnel: i32[] [1310, 1490, 1550, 1625] -> [w364]
          tunnel: w336 -> [w361]
          tunnel: w354 -> [w359]
          shift-right: [w363] -> w349
          shift-left: w337 -> [w360]
          tunnel: w352 -> [w358] mode=indexing
          tunnel: [w356] -> w347
          i -> [w362]
          n122 = Increment(x=w362) -> (x+1=w357:i32)
          n123 = case shown="True" w358 {
            tunnel: w364 -> [_ w377]
            tunnel: [w366 w376] -> w363
            tunnel: w361 -> [w365 w375]
            tunnel: w360 -> [w366 w373]
            tunnel: w359 -> [_ w370]
            tunnel: w357 -> [_ w367]
            tunnel: [w365 w368] -> w356
            frame False {
            }
            frame True {
              n124 = Array Size(array=w370) -> (size(s)=w369:i32)
              n125 = call "Enqueue Message.vi"("error in (no error)"=w373, "Message Data"=w367, "Message"="device:switch", "Message Queue"=w375) -> ("error out"=w372:errorcluster, "dup Message Queue"=w374:refnum<queue>)  [unwired: 6 in]
              n126 = for "Wavelength Loop" {
                N: w369 -> [_]
                tunnel: w370 -> [w390] mode=indexing
                tunnel: w377 -> [w389] mode=indexing
                tunnel: w374 -> [w388]
                shift-right: [w381] -> w376
                shift-left: w372 -> [w387]
                tunnel: [w382] -> w368
                n127 = case shown="True" w390 {
                  selector: w390 -> [w393 w395]
                  tunnel: w389 -> [_ w398]
                  tunnel: w388 -> [w392 w399]
                  tunnel: [w391 w397] -> w386
                  tunnel: [w392 w396] -> w385
                  tunnel: [w393 w395] -> w384
                  tunnel: w387 -> [w391 w394]
                  frame False {
                  }
                  frame True {
                    n128 = call "Enqueue Message.vi"("error in (no error)"=w394, "Message Data"=w398, "Message"="device:reference", "Message Queue"=w399) -> ("error out"=w397:errorcluster, "dup Message Queue"=w396:refnum<queue>)  [unwired: 6 in]
                  }
                }
                n129 = call "Enqueue Message.vi"("error in (no error)"=w386, "Message Data"=w384, "Message"="device:getRefData", "Message Queue"=w385) -> ("error out"=w378:errorcluster, "dup Message Queue"=w379:refnum<queue>)  [unwired: 6 in]
                n130 = call "Enqueue Message.vi"("error in (no error)"=w378, "Message"="data:buildTable", "Message Queue"=w379) -> ("error out"=w381:errorcluster, "dup Message Queue"=w382:refnum<queue>)  [unwired: 7 in]
              }
            }
          }
        }
        n131 = call "Enqueue Message.vi"("error in (no error)"=w349, "Message"="UI:endSubstRef", "Message Queue"=w347) -> ("error out"=w348:errorcluster)  [unwired: 7 in, 1 out]
      }
      frame "macro:queueMeas" {
        # "Queues the messages necessary for measurements and dataGets for each selected wavelength per channel"
        n132 = Unbundle By Name(w409) -> ("Viavi - objectRefs.ChannelRef"=w402:refnum<vi>, "Viavi - objectRefs.WavelengthRef"=w401:refnum<vi>)
        n133 = property class="Arr (strict)"(reference=w401, error in=w410) -> ("Value"=w411:bool[])  [unwired: 2 out]
        n134 = property class="Arr (strict)"(reference=w402, error in=w410) -> ("Value"=w408:bool[])  [unwired: 2 out]
        n135 = Array Size(array=w408) -> (size(s)=w407:i32)
        n136 = for "Channel Loop" {
          N: w407 -> [_]
          tunnel: i32[] [1310, 1490, 1550, 1625] -> [w422]
          tunnel: w413 -> [w419]
          tunnel: w411 -> [w417]
          shift-right: [w421] -> w405
          shift-left: w410 -> [w418]
          tunnel: w408 -> [w416] mode=indexing
          tunnel: [w414] -> w403
          i -> [w420]
          n137 = Increment(x=w420) -> (x+1=w415:i32)
          n138 = case shown="True" w416 {
            tunnel: w422 -> [_ w435]
            tunnel: [w424 w434] -> w421
            tunnel: w419 -> [w423 w433]
            tunnel: w418 -> [w424 w431]
            tunnel: w417 -> [_ w428]
            tunnel: w415 -> [_ w425]
            tunnel: [w423 w426] -> w414
            frame False {
            }
            frame True {
              n139 = Array Size(array=w428) -> (size(s)=w427:i32)
              n140 = call "Enqueue Message.vi"("error in (no error)"=w431, "Message Data"=w425, "Message"="device:switch", "Message Queue"=w433) -> ("error out"=w430:errorcluster, "dup Message Queue"=w432:refnum<queue>)  [unwired: 6 in]
              n141 = for "Wavelength Loop" {
                N: w427 -> [_]
                tunnel: w428 -> [w448] mode=indexing
                tunnel: w435 -> [w447] mode=indexing
                tunnel: w432 -> [w446]
                shift-right: [w439] -> w434
                shift-left: w430 -> [w445]
                tunnel: [w440] -> w426
                n142 = case shown="True" w448 {
                  selector: w448 -> [w451 w453]
                  tunnel: w447 -> [_ w456]
                  tunnel: w446 -> [w450 w457]
                  tunnel: [w449 w455] -> w444
                  tunnel: [w450 w454] -> w443
                  tunnel: [w451 w453] -> w442
                  tunnel: w445 -> [w449 w452]
                  frame False {
                  }
                  frame True {
                    n143 = call "Enqueue Message.vi"("error in (no error)"=w452, "Message Data"=w456, "Message"="device:measure", "Message Queue"=w457) -> ("error out"=w455:errorcluster, "dup Message Queue"=w454:refnum<queue>)  [unwired: 6 in]
                  }
                }
                n144 = call "Enqueue Message.vi"("error in (no error)"=w444, "Message Data"=w442, "Message"="device:getMeasData", "Message Queue"=w443) -> ("error out"=w436:errorcluster, "dup Message Queue"=w437:refnum<queue>)  [unwired: 6 in]
                n145 = call "Enqueue Message.vi"("error in (no error)"=w436, "Message"="data:buildTable", "Message Queue"=w437) -> ("error out"=w439:errorcluster, "dup Message Queue"=w440:refnum<queue>)  [unwired: 7 in]
              }
            }
          }
        }
        n146 = call "Enqueue Message.vi"("error in (no error)"=w405, "Message"="UI:endMeas", "Message Queue"=w403) -> ("error out"=w404:errorcluster)  [unwired: 7 in, 1 out]
      }
      frame "macro:instructions" {
        # "Multichannel\n8: Take reference\n9: Take reference (substitution)\n10: Take reference (cutback)\n11: Measure DUT\n12: Measure DUT (substitution)\n13: Measure DUT (cutback)"
        # "Instruction indexes:\n0: Take reference\n1: Take reference (substitution)\n2: Take reference (cutback)\n3: Measure DUT\n4: Measure DUT (substitution)\n5: Measure DUT (cutback)\n6: Disconnect Integrating Sphere\n7: Connect Integrating Sphere"
        # "Opens the instruction tab and sets the text and image\nCalls instructWait to pause program until user clicks ok\nRequires index of desired instruction display\nChange Instructions control to add new instructions"
        n147 = Variant To Data(error in=w479, type=0, Variant=w478) -> (data=w465:i32, error out=w471:errorcluster)
        n148 = Cluster To Array(cluster=T17 {"Reference Instructions"={"Instruction Text"="Connect launch cable to power meter.\nClick OK when step completed.", "Instruction Image"=bytes[542649], "Main Display Message"="Referencing"}, "Reference (substitution) Instructions"={"Instruction Text"="Connect launch cable to recieve cable, and recieve cable to power meter.\nClick OK when step completed.", "Instruction Image"=bytes[542649], "Main Display Message"="Referencing"}, "Reference (cutback) Instructions"={"Instruction Text"="Connect launch cable to power meter.\nClick OK when step completed.", "Instruction Image"=bytes[542649], "Main Display Message"="Referencing"}, "Measure Instructions"={"Instruction Text"="Connect launch cable to DUT, and DUT to power meter.\nClick OK when step completed.", "Instruction Image"=bytes[544350], "Main Display Message"="Measuring"}, "Measure (Substitution) Instructions"={"Instruction Text"="Connect launch cable to DUT, DUT to recieve cable, and recieve cable to power meter.\nClick OK when step completed.", "Instruction Image"=bytes[526395], "Main Display Message"="Measuring"}, "Measure (Cutback) Instructions"={"Instruction Text"="Connect launch cable to DUT, and DUT to power meter.\nClick OK when step completed.", "Instruction Image"=bytes[544350], "Main Display Message"="Measuring"}, "Disconnect Int Sphere Instructions"={"Instruction Text"="Disconnect integrating sphere and connect launch cable to power meter\nClick OK when step completed.", "Instruction Image"=bytes[612030], "Main Display Message"="Measuring pRatio"}, "Connect Int Sphere Instructions"={"Instruction Text"="Connect integrating sphere and connect launch cable to integrating sphere.\nClick OK when step completed.", "Instruction Image 2"=bytes[612030], "Main Display Message"="Measuring pRatio"}, " Multichannel Reference Instructions"={"Instruction Text"="Connect launch cable to power meter.\nClick OK when step completed.", "Instruction Image"=bytes[542649], "Main Display Message"="Referencing"}, " Multichannel Reference (substitution) Instructions"={"Instruction Text"="Connect launch cable to recieve cable, and recieve cable to power meter.\nClick OK when step completed.", "Instruction Image"=bytes[542649], "Main Display Message"="Referencing"}, " Multichannel Reference (cutback) Instructions"={"Instruction Text"="Connect launch cable to power meter.\nClick OK when step completed.", "Instruction Image"=bytes[542649], "Main Display Message"="Referencing"}, "Multichannel Measure Instructions"={"Instruction Text"="Connect launch cable to DUT, and DUT to power meter.\nClick OK when step completed.", "Instruction Image"=bytes[537345], "Main Display Message"="Measuring"}, "Multichannel Measure (Substitution) Instructions"={"Instruction Text"="Connect launch cable to DUT, and DUT to power meter.\nClick OK when step completed.", "Instruction Image"=bytes[537345], "Main Display Message"="Measuring"}, "Multichannel Measure (Cutback) Instructions"={"Instruction Text"="Connect launch cable to DUT, and DUT to power meter.\nClick OK when step completed.", "Instruction Image"=bytes[537345], "Main Display Message"="Measuring"}} ("Instructions")) -> (array=w467:T23)
        n149 = Index Array(array=w467, index=w465) -> (element=w464:T24)
        n150 = Unbundle By Name(w464) -> ("Instruction Text"=→"Instruction Text":string, "Instruction Image"=→"Instruction Image":picture, "Main Display Message"=w463:string)
        n151 = Unbundle By Name(w462) -> ("Viavi - objectRefs.instructButtonRef"=w461:refnum<vi>)
        n152 = property class="Bool"(reference=w461, "DisabledEnum"=T14."Enabled" ("Disabled")) -> ()  [unwired: 1 in, 2 out]
        n153 = call "Enqueue Message.vi"("Priority Message? (F)"=TRUE, "error in (no error)"=w471, "Message Data"=w463, "Message"="macro:instructWait", "Message Queue"=w470) -> ("error out"=w468:errorcluster, "dup Message Queue"=w469:refnum<queue>)  [unwired: 5 in]
        n154 = call "Enqueue Message.vi"("Priority Message? (F)"=TRUE, "error in (no error)"=w468, "Message Data"=2, "Message"="UI:setTab", "Message Queue"=w469) -> ("error out"=w474:errorcluster)  [unwired: 5 in, 1 out]
      }
      frame "macro:instructWait" {
        # "Waits until the user has clicked the instruction ok button"
        n155 = case shown="True" "Instruction Button" {
          tunnel: [w494 w505] -> w486
          tunnel: w488 -> [_ w509]
          tunnel: w483 -> [w502 w507]
          tunnel: w485 -> [w500 _]
          tunnel: w484 -> [w501 w503]
          tunnel: w482 -> [w489 _]
          frame True {
            n156 = Variant To Data(error in=w502, type="", Variant=w501) -> (data=w499:string, error out=w496:errorcluster)
            n157 = Unbundle By Name(w489) -> ("Viavi - objectRefs.instructButtonRef"=w491:refnum<vi>)
            n158 = call "Enqueue Message.vi"("error in (no error)"=w496, "Message Data"=w499, "Message"="UI:updateDisplay", "Message Queue"=w500) -> ("error out"=w495:errorcluster, "dup Message Queue"=w493:refnum<queue>)  [unwired: 6 in]
            n159 = property class="Bool"(reference=w491, "DisabledEnum"=T14."Disabled and Grayed Out" ("Disabled")) -> ()  [unwired: 1 in, 2 out]
            n160 = call "Enqueue Message.vi"("error in (no error)"=w495, "Message"="UI:startRun", "Message Queue"=w493) -> ("error out"=w494:errorcluster)  [unwired: 7 in, 1 out]
          }
          frame False {
            n161 = call "Enqueue Message.vi"("Priority Message? (F)"=TRUE, "error in (no error)"=w507, "Message Data"=w503, "Message"="macro:instructWait", "Message Queue"=w509) -> ("error out"=w506:errorcluster)  [unwired: 5 in, 1 out]
            n162 = call "Stall Data Flow.vim"("value in"=w506, "milliseconds to wait"=u32 500) -> ("value out"=w505:errorcluster)  [unwired: 1 out]
          }
        }
      }
      frame "macro:preset" {
        # "Sets the RL Configs based on the selected RL Preset or custom settings"
        n163 = Unbundle By Name(w513) -> ("Viavi - objectRefs.RLPresetRef"=w511:refnum<vi>)
        n164 = control-ref of="Custom RL Cluster"() -> (w514:refnum<vi>)
        n165 = property class="RadioBtnsControl (strict)"(reference=w511) -> ("Value"=w512:T5)  [unwired: 1 in, 2 out]
        n166 = case shown="\"Custom\", Default" w512 {
          tunnel: [T6 {"Measurement Mode"=FALSE, "Enable RL2"=FALSE, "RL1 Anchor Point"=enum."Left DUT Connection", "RL1 Measure Points"={-0.2500000000000009, 0.25}, "RL2 Anchor Point"=enum."Right DUT Connection", "RL2 Measure Points"={-0.2500000000000009, 0.25}} ("RL Configs") T6 {"Measurement Mode"=FALSE, "Enable RL2"=FALSE, "RL1 Anchor Point"=enum."Right DUT Connection", "RL1 Measure Points"={-0.2500000000000009, 0.25}, "RL2 Anchor Point"=enum."Right DUT Connection", "RL2 Measure Points"={-0.2500000000000009, 0.25}} ("RL Configs") T6 {"Measurement Mode"=TRUE, "Enable RL2"=FALSE, "RL1 Anchor Point"=enum."Center on DUT", "RL1 Measure Points"={-0.5, 0.5}, "RL2 Anchor Point"=enum."Right DUT Connection", "RL2 Measure Points"={-0.2500000000000009, 0.25}} ("RL Configs") T6 {"Measurement Mode"=FALSE, "Enable RL2"=TRUE, "RL1 Anchor Point"=enum."Left DUT Connection", "RL1 Measure Points"={-0.2500000000000009, 0.25}, "RL2 Anchor Point"=enum."Right DUT Connection", "RL2 Measure Points"={-0.2500000000000009, 0.25}} ("RL Configs") w555] -> w520
          tunnel: w515 -> [_ _ _ _ _]
          tunnel: [w526 w530 w534 w538 w557] -> w516
          tunnel: w517 -> [w526 w530 w534 w538 w557]
          tunnel: w514 -> [w525 w528 w532 w536 _]
          frame "Left Anchor" {
            n167 = property class="Clust (strict)"(reference=w525, "Value"=T4 {"Enable Integral"=FALSE, "RL 1 A"=0.0, "RL 1 B"=0.0, "RL 2 A"=0.0, "RL 2 B"=0.0, "Enable RL2"=FALSE, "RL Method"=0} ("Custom RL Cluster")) -> ()  [unwired: 1 in, 2 out]
          }
          frame "Right Anchor" {
            n168 = property class="Clust (strict)"(reference=w528, "Value"=T4 {"Enable Integral"=FALSE, "RL 1 A"=0.0, "RL 1 B"=0.0, "RL 2 A"=0.0, "RL 2 B"=0.0, "Enable RL2"=FALSE, "RL Method"=0} ("Custom RL Cluster")) -> ()  [unwired: 1 in, 2 out]
          }
          frame "Center Anchor" {
            n169 = property class="Clust (strict)"(reference=w532, "Value"=T4 {"Enable Integral"=FALSE, "RL 1 A"=0.0, "RL 1 B"=0.0, "RL 2 A"=0.0, "RL 2 B"=0.0, "Enable RL2"=FALSE, "RL Method"=0} ("Custom RL Cluster")) -> ()  [unwired: 1 in, 2 out]
          }
          frame "Left/Right Anchor" {
            n170 = property class="Clust (strict)"(reference=w536, "Value"=T4 {"Enable Integral"=FALSE, "RL 1 A"=0.0, "RL 1 B"=0.0, "RL 2 A"=0.0, "RL 2 B"=0.0, "Enable RL2"=FALSE, "RL Method"=0} ("Custom RL Cluster")) -> ()  [unwired: 1 in, 2 out]
          }
          frame "Custom", Default {
            n171 = Unbundle By Name("Custom RL Cluster") -> ("Enable Integral"=w546:bool, "Enable RL2"=w545:bool, "RL Method"=w542:u16, "RL 1 A"=w553:dbl, "RL 1 B"=w552:dbl, "RL 2 A"=w551:dbl, "RL 2 B"=w550:dbl)
            n172 = Not Equal?(x=w542, y=4) -> (x != y?=w543:bool)
            n173 = Select(t=w542, s=w543, f=1) -> (s? t:f=w541:i32)
            n174 = Bundle("RL 1 A"=w553, "RL 1 B"=w552) -> (w548:cluster{"RL 1 A":dbl, "RL 1 B":dbl})  [unwired: 1 in]
            n175 = Bundle("RL 2 A"=w551, "RL 2 B"=w550) -> (w549:cluster{"RL 2 A":dbl, "RL 2 B":dbl})  [unwired: 1 in]
            n176 = Bundle By Name(cluster=T6 {"Measurement Mode"=FALSE, "Enable RL2"=FALSE, "RL1 Anchor Point"=enum."Left DUT Connection", "RL1 Measure Points"={-0.2500000000000009, 0.25}, "RL2 Anchor Point"=enum."Right DUT Connection", "RL2 Measure Points"={-0.2500000000000009, 0.25}} ("RL Configs"), "Measurement Mode"=w546, "Enable RL2"=w545, "RL1 Anchor Point"=w541, "RL1 Measure Points"=w548, "RL2 Anchor Point"=2, "RL2 Measure Points"=w549) -> (w555:T6)
          }
        }
        "RL Configs" <- w520
        n177 = Unbundle By Name(w513) -> ("Viavi - objectRefs.RL2StandardRef"=w523:refnum<vi>)
        n178 = Unbundle By Name(w520) -> ("Enable RL2"=w521:bool)
        n179 = Select(t=0, s=w521, f=2) -> (s? t:f=w522:i32)
        n180 = property class="Ring (strict)"(reference=w523, "DisabledEnum"=w522) -> ()  [unwired: 1 in, 2 out]
      }
      frame "---------- Core ----------" {
        # "Template Separator\n(You can make a copy of, or modify, this frame)"
      }
      frame Default {
        # "'Default' case only runs if there is a message that isn't defined in any of the other cases.  Output a programming error."
        n181 = xnode "Error Ring"("parameter 0"=w560) -> ("error out"=w561:errorcluster)
      }
      frame "core:error" {
        # "To igonore errors:\n\nadd error code as a case statement and clear the error."
        # "Send error cluster to MHL to log to Error Log.txt, generate a user error dialog, and clear error."
        n182 = Variant To Data(error in=w576, type=errorcluster {"status"=FALSE, "code"=0, "source"=""} ("error out"), Variant=w575) -> (data=w579:errorcluster, error out=w578:errorcluster)
        n183 = Merge Errors(w579, w578) -> (w573:errorcluster)
        n184 = Unbundle By Name(w573) -> ("code"=w574:i32)
        n185 = case "Send or Ignore Error" shown="Default" w574 {
          tunnel: w573 -> [w583]
          tunnel: w572 -> [_]
          tunnel: [w588] -> w571
          tunnel: w570 -> [w587]
          frame Default {
            # "Propagate error up to MHL. Send status message to MHL."
            n186 = To Variant(anything=w583) -> (Variant=w581:variant)
            n187 = To Variant(anything="Error in SubVI.") -> (Variant=w582:variant)
            n188 = Build Array(w581, w582) -> (w584:variant[])
            n189 = call "sendMultipleMessages.vi"("messageData"=w584, "queueMessages"=T13 [{"queueName"="MHL", "queueMessage"="core:error", "priority?"=FALSE}, {"queueName"="MHL", "queueMessage"="UI:updateDisplay", "priority?"=FALSE}], "messageQueues"=w587) -> ("error out"=w588:errorcluster)  [unwired: 8 in]
          }
        }
      }
      frame "core:exit" {
        w596 = TRUE  # notification
        # "Release queue, Fire user Stop event to shutdown UI loop, and send exit notification to MHL."
        n190 = Release Queue(queue=w599, error in (no error)=w595) -> (error out=w593:errorcluster)  [unwired: 1 in, 2 out]
        n191 = Unbundle By Name(w590) -> ("stop"=w589:refnum<user-event>)
        n192 = call "fireEventStop.vi"("error in (no error)"=w593, "stop"=w589) -> ("error out"=w592:errorcluster)  [unwired: 9 in]
        n193 = Send Notification(notification=w596, notifier=w597, error in (no error)=w592) -> (error out=w591:errorcluster)  [unwired: 1 out]
      }
      frame "---------- Data ----------" {
        # "Template Separator\n(You can make a copy of, or modify, this frame)"
      }
      frame "data:cleanRefTemps" {
        w603 = T2 [] ("Value")
        # "Removes all values from the current reference arrays"
        n194 = Unbundle By Name(w605) -> ("Viavi - objectRefs.TempRefPowRef"=w606:refnum<vi>, "Viavi - objectRefs.RefLengthRef"=w602:refnum<vi>)
        n195 = property class="Arr (strict)"(reference=w606, error in=w604, "Value"=w603) -> ()  [unwired: 2 out]
        n196 = property class="Arr (strict)"(reference=w602, error in=w604, "Value"=w603) -> ()  [unwired: 2 out]
      }
      frame "data:cleanMeasTemps" {
        w607 = T2 [] ("Value")
        # "Removes all values from the current reference arrays"
        n197 = Unbundle By Name(w614) -> ("Viavi - objectRefs.TempILRef"=w609:refnum<vi>, "Viavi - objectRefs.TempRLRef"=w613:refnum<vi>, "Viavi - objectRefs.TempRL2Ref"=w610:refnum<vi>, "Viavi - objectRefs.TempPowRef"=w612:refnum<vi>, "Viavi - objectRefs.LengthArrayRef"=w611:refnum<vi>)
        n198 = property class="Arr (strict)"(reference=w609, error in=w608, "Value"=w607) -> ()  [unwired: 2 out]
        n199 = property class="Arr (strict)"(reference=w613, error in=w608, "Value"=w607) -> ()  [unwired: 2 out]
        n200 = property class="Arr (strict)"(reference=w610, error in=w608, "Value"=w607) -> ()  [unwired: 2 out]
        n201 = property class="Arr (strict)"(reference=w612, error in=w608, "Value"=w607) -> ()  [unwired: 2 out]
        n202 = property class="Arr (strict)"(reference=w611, error in=w608, "Value"=w607) -> ()  [unwired: 2 out]
      }
      frame "data:buildTable" {
        # "Builds the single channel or multi channel tables used as data visualization"
        n203 = Unbundle By Name(w633) -> ("Viavi - objectRefs.SingleChannelRef"=w625:refnum<vi>, "Viavi - objectRefs.TempRefPowRef"=w624:refnum<vi>, "Viavi - objectRefs.TempILRef"=w623:refnum<vi>, "Viavi - objectRefs.TempRLRef"=w622:refnum<vi>, "Viavi - objectRefs.TempRL2Ref"=w621:refnum<vi>, "Viavi - objectRefs.ChannelRef"=w620:refnum<vi>)
        n204 = property class="Bool (strict)"(reference=w625, error in=w617) -> ("Value"=w629:bool)  [unwired: 2 out]
        n205 = property class="Arr (strict)"(reference=w624, error in=w617) -> ("Value"=w632:T2)  [unwired: 2 out]
        n206 = property class="Arr (strict)"(reference=w623, error in=w617) -> ("Value"=w631:T2)  [unwired: 2 out]
        n207 = property class="Arr (strict)"(reference=w622, error in=w617) -> ("Value"=w630:T2)  [unwired: 2 out]
        n208 = property class="Arr (strict)"(reference=w621, error in=w617) -> ("Value"=w626:T2)  [unwired: 2 out]
        n209 = property class="Arr (strict)"(reference=w620, error in=w617) -> ("Value"=w627:bool[])  [unwired: 2 out]
        n210 = Bundle(cluster=T18 {"Temp Ref Power Array"=[], "Temp IL Array"=[], "Temp RL Array"=[], "Temp RL2 Array"=[]} ("Data Input"), "Temp Ref Power Array"=w632, "Temp IL Array"=w631, "Temp RL Array"=w630, "Temp RL2 Array"=w626) -> (w628:T18)
        n211 = case shown="False" w629 {
          tunnel: w628 -> [w636 w639]
          tunnel: [_ w638] -> w618
          tunnel: [w635 _] -> w615
          tunnel: w627 -> [w637 _]
          tunnel: [w634 _] -> w616
          frame False {
            n212 = call "Viavi - Multi Channel Table.vi"("Channels Selected"=w637, "Data Input"=w636) -> ("RL Table Output"=w634:T7, "Ref IL Table Output"=w635:T7)  [unwired: 7 in]
          }
          frame True {
            n213 = call "Viavi - Single Channel Table.vi"("Data Input"=w639) -> ("Table Output"=w638:T7)  [unwired: 10 in]
          }
        }
        "Single Table" <- w618
        "Multi Ref/IL Table" <- w615
        "Multi RL Table" <- w616
      }
      frame "data:sendSaveData" {
        # "Sends the current temp data to the main VI to save\nSends the optional save data as RL2 to location 3 of save"
        n214 = Unbundle By Name(w668) -> ("Viavi - objectRefs.TempILRef"=w667:refnum<vi>, "Viavi - objectRefs.TempRLRef"=w665:refnum<vi>, "Viavi - objectRefs.TempRefPowRef"=w666:refnum<vi>, "Viavi - objectRefs.TempPowRef"=w664:refnum<vi>, "Viavi - objectRefs.TempRL2Ref"=w663:refnum<vi>, "Viavi - objectRefs.RLConfigsRef"=w662:refnum<vi>)
        n215 = property class="Arr (strict)"(reference=w667, error in=w658) -> ("Value"=w642:T2)  [unwired: 2 out]
        n216 = property class="Arr (strict)"(reference=w665, error in=w658) -> ("Value"=w661:T2)  [unwired: 2 out]
        n217 = property class="Arr (strict)"(reference=w666, error in=w658) -> ("Value"=w660:T2)  [unwired: 2 out]
        n218 = property class="Arr (strict)"(reference=w664, error in=w658) -> ("Value"=w659:T2)  [unwired: 2 out]
        n219 = property class="Arr (strict)"(reference=w663, error in=w658) -> ("Value"=w641:T2)  [unwired: 2 out]
        n220 = property class="Clust (strict)"(reference=w662, error in=w658) -> ("Value"=w669:T22)  [unwired: 2 out]
        n221 = for {
          tunnel: w642 -> [w692] mode=indexing
          tunnel: w661 -> [w691] mode=indexing
          tunnel: w660 -> [w690] mode=indexing
          tunnel: w659 -> [w689] mode=indexing
          tunnel: [w680] -> w651 mode=indexing
          tunnel: [w679] -> w652 mode=indexing
          tunnel: [w678] -> w653 mode=indexing
          tunnel: [w677] -> w654 mode=indexing
          n222 = call "Viavi - prepSave.vi"("Decimal Points"=3, "Input Data"=w692) -> ("Fail"=w683:bool, "Data Output"=w684:string)  [unwired: 8 in]
          n223 = call "Viavi - prepSave.vi"("Decimal Points"=2, "Input Data"=w691) -> ("Fail"=w681:bool, "Data Output"=w682:string)  [unwired: 8 in]
          n224 = call "Viavi - prepSave.vi"("Decimal Points"=3, "Input Data"=w690) -> ("Data Output"=w679:string)  [unwired: 8 in, 1 out]
          n225 = call "Viavi - prepSave.vi"("Decimal Points"=3, "Input Data"=w689) -> ("Data Output"=w680:string)  [unwired: 8 in, 1 out]
          n226 = Bundle("Data Output"=w684, "Fail"=w683) -> (w677:cluster{"Data Output":string, "Fail":bool})  [unwired: 1 in]
          n227 = Bundle("Data Output"=w682, "Fail"=w681) -> (w678:cluster{"Data Output":string, "Fail":bool})  [unwired: 1 in]
        }
        n228 = for {
          tunnel: w641 -> [w673] mode=indexing
          tunnel: [w672] -> w640 mode=indexing
          n229 = call "Viavi - prepSave.vi"("Decimal Points"=2, "Input Data"=w673) -> ("Fail"=w676:bool, "Data Output"=w675:string)  [unwired: 8 in]
          n230 = Bundle("Data Output"=w675, "Fail"=w676) -> (w672:cluster{"Data Output":string, "Fail":bool})  [unwired: 1 in]
        }
        n231 = Unbundle By Name(w669) -> ("Enable RL2"=w656:bool)
        n232 = Select(t=w640, s=w656, f=cluster{"Data Output":string, "Fail":bool}[] []) -> (s? t:f=w650:cluster{"Data Output":string, "Fail":bool}[])
        n233 = Bundle(cluster=T19 {"IL Array"=[], "RL Array"=[], "Ref Power Array"=[], "Power Array"=[], "Optional Data Array"=[], "Optional Param"=""}, "IL Array"=w654, "RL Array"=w653, "Ref Power Array"=w652, "Power Array"=w651, "Optional Data Array"=w650, "Optional Param"="RL 2 Parameter") -> (w657:T19)
        n234 = call "Enqueue Message.vi"("error in (no error)"=w658, "Message Data"=w657, "Message"="data:saveData", "Message Queue"=w671) -> ("error out"=w645:errorcluster, "dup Message Queue"=w644:refnum<queue>)  [unwired: 6 in]
        n235 = call "Enqueue Message.vi"("error in (no error)"=w645, "Message Data"="Data saved" ("Message"), "Message"="UI:updateDisplay", "Message Queue"=w644) -> ("error out"=w643:errorcluster)  [unwired: 6 in, 1 out]
      }
      frame "---------- UI ----------" {
        # "Template Separator\n(You can make a copy of, or modify, this frame)"
      }
      frame "UI:initConfig" {
        # "Initializes the SubVI configs when a new test occurs"
        n236 = Unbundle By Name(w710) -> ("Viavi - objectRefs.RL2StandardRef"=w709:refnum<vi>, "Viavi - objectRefs.RLConfigsRef"=w715:refnum<vi>, "Viavi - objectRefs.RLPresetRef"=w703:refnum<vi>, "Viavi - objectRefs.instructButtonRef"=w702:refnum<vi>)
        n237 = control-ref of="First Reference"() -> (w714:refnum<vi>)
        n238 = call "IL-RL Standards.vi"("Input New Standard"=T20 {"Standard Name"="", "Max IL to Pass (dB)"=0.0, "Min RL to Pass (dB)"=0.0}) -> ("Standard Names"=w706:string[])  [unwired: 8 in, 1 out]
        n239 = Replace Array Subset(array=w706, new element="Select RL2 Standard" ("new element/subarray"), index=0) -> (w707:string[])
        n240 = property class="Ring (strict)"(reference=w709, "Value"=u16 0, "Strings []"=w707) -> ()  [unwired: 1 in, 2 out]
        n241 = property class="Clust (strict)"(reference=w715, "Value"=T6 {"Measurement Mode"=FALSE, "Enable RL2"=FALSE, "RL1 Anchor Point"=enum."Left DUT Connection", "RL1 Measure Points"={-0.2500000000000009, 0.25}, "RL2 Anchor Point"=enum."Right DUT Connection", "RL2 Measure Points"={-0.2500000000000009, 0.25}} ("RL Configs")) -> ()  [unwired: 1 in, 2 out]
        n242 = property class="RadioBtnsControl (strict)"(reference=w703, "Value"=T5."Left Anchor") -> ()  [unwired: 1 in, 2 out]
        n243 = property class="Bool"(reference=w702, "DisabledEnum"=T14."Enabled" ("Disabled")) -> ()  [unwired: 1 in, 2 out]
        n244 = property class="Bool (strict)"(reference=w714, "Value"=TRUE) -> ()  [unwired: 1 in, 2 out]
        n245 = call "Enqueue Message.vi"("error in (no error)"=w699, "Message Data"=FALSE ("Value"), "Message"="UI:disableRL", "Message Queue"=w697) -> ("error out"=w698:errorcluster)  [unwired: 6 in, 1 out]
      }
      frame "UI:disableRL" {
        # "Disables the RL options when RL is not enabled"
        n246 = Variant To Data(error in=w729, type=TRUE, Variant=w728) -> (data=w726:bool, error out=w722:errorcluster)
        n247 = Select(t=T14."Enabled" ("Disabled"), s=w726, f=T14."Disabled and Grayed Out" ("Disabled")) -> (s? t:f=w716:T14)
        n248 = Unbundle By Name(w723) -> ("Viavi - objectRefs.RLPresetRef"=w731:refnum<vi>, "Viavi - objectRefs.RLConfigsRef"=w730:refnum<vi>)
        n249 = control-ref of="Input Image"() -> (w718:refnum<vi>)
        n250 = control-ref of="Output Image"() -> (w719:refnum<vi>)
        n251 = control-ref of="Between Image"() -> (w720:refnum<vi>)
        n252 = control-ref of="Both Image"() -> (w721:refnum<vi>)
        n253 = control-ref of="Custom RL Cluster"() -> (w717:refnum<vi>)
        n254 = property class="RadioBtnsControl (strict)"(reference=w731, "DisabledEnum"=w716) -> ()  [unwired: 1 in, 2 out]
        n255 = property class="Clust (strict)"(reference=w730, "DisabledEnum"=w716) -> ()  [unwired: 1 in, 2 out]
        n256 = property class="Pict"(reference=w718, "DisabledEnum"=w716) -> ()  [unwired: 1 in, 2 out]
        n257 = property class="Pict"(reference=w719, "DisabledEnum"=w716) -> ()  [unwired: 1 in, 2 out]
        n258 = property class="Pict"(reference=w720, "DisabledEnum"=w716) -> ()  [unwired: 1 in, 2 out]
        n259 = property class="Pict"(reference=w721, "DisabledEnum"=w716) -> ()  [unwired: 1 in, 2 out]
        n260 = property class="Clust (strict)"(reference=w717, "DisabledEnum"=w716) -> ()  [unwired: 1 in, 2 out]
      }
      frame "UI:endRef" {
        # "Sets UI state to reference end\nIf in substitution mode begins the sequence for taking the second measurement"
        n261 = Unbundle By Name(w740) -> ("Viavi - objectRefs.MethodSelectRef"=w739:refnum<vi>, "Viavi - objectRefs.SingleChannelRef"=w735:refnum<vi>)
        n262 = property class="Ring (strict)"(reference=w739) -> ("Value"=w738:u16)  [unwired: 1 in, 2 out]
        n263 = property class="Bool (strict)"(reference=w735) -> ("Value"=w734:bool)  [unwired: 1 in, 2 out]
        n264 = call "Enqueue Message.vi"("error in (no error)"=w744, "Message Data"="Reference completed", "Message"="UI:updateDisplay", "Message Queue"=w743) -> ("error out"=w737:errorcluster, "dup Message Queue"=w732:refnum<queue>)  [unwired: 6 in]
        n265 = case shown="Default" w738 {
          tunnel: w733 -> [w745 _]
          tunnel: w737 -> [w749 w765]
          tunnel: [w750 w763] -> w736
          tunnel: w734 -> [w755 _]
          tunnel: w732 -> [w748 w766]
          frame 3 {
            n266 = call "Enqueue Message.vi"("error in (no error)"=w749, "Message"="UI:endRun", "Message Queue"=w748) -> ("error out"=w746:errorcluster)  [unwired: 7 in, 1 out]
            n267 = Select(t=1, s=w755, f=9) -> (s? t:f=w754:i32)
            n268 = call "Enqueue Message.vi"("error in (no error)"=w746, "Message Data"=w754, "Message"="macro:instructions", "Message Queue"=w745) -> ("error out"=w759:errorcluster, "dup Message Queue"=w760:refnum<queue>)  [unwired: 6 in]
            n269 = call "Enqueue Message.vi"("error in (no error)"=w759, "Message Data"=1, "Message"="UI:setTab", "Message Queue"=w760) -> ("error out"=w751:errorcluster, "dup Message Queue"=w752:refnum<queue>)  [unwired: 6 in]
            n270 = call "Enqueue Message.vi"("error in (no error)"=w751, "Message"="macro:queueSubstRef", "Message Queue"=w752) -> ("error out"=w750:errorcluster)  [unwired: 7 in, 1 out]
          }
          frame Default {
            n271 = call "Enqueue Message.vi"("error in (no error)"=w765, "Message"="UI:endRef", "Message Queue"=w766) -> ("error out"=w763:errorcluster)  [unwired: 7 in, 1 out]
          }
        }
      }
      frame "UI:endMeas" {
        # "Sets UI state to measure end\nWhen a length value error is received reset to end reference state\nWhen an failure occurs, uses the failure message rather then measurement complete"
        n272 = Unbundle By Name(w770) -> ("Viavi - objectRefs.DataErrorRef"=w769:refnum<vi>)
        n273 = property class="Str"(reference=w769) -> ("Value"=w767:string)  [unwired: 1 in, 2 out]
        n274 = case shown="\"Length unknown. Retest required. Dirty connector or incorrect cable.\"" w767 {
          tunnel: w777 -> [w782 w787]
          tunnel: w776 -> [w781 w786]
          tunnel: [w780 w785] -> w775
          tunnel: [w779 w784] -> w774
          frame Default {
            n275 = call "Enqueue Message.vi"("error in (no error)"=w782, "Message"="UI:endMeas", "Message Queue"=w781) -> ("error out"=w780:errorcluster, "dup Message Queue"=w779:refnum<queue>)  [unwired: 7 in]
          }
          frame "Length unknown. Retest required. Dirty connector or incorrect cable." {
            n276 = call "Enqueue Message.vi"("error in (no error)"=w787, "Message"="UI:endRef", "Message Queue"=w786) -> ("error out"=w785:errorcluster, "dup Message Queue"=w784:refnum<queue>)  [unwired: 7 in]
          }
        }
        n277 = Empty String/Path?(string/path=w767) -> (empty?=w768:bool)
        n278 = case shown="True" w768 {
          tunnel: [w788 "Measurement complete"] -> w773
          tunnel: w767 -> [w788 _]
          frame False {
          }
          frame True {
          }
        }
        n279 = call "Enqueue Message.vi"("error in (no error)"=w775, "Message Data"=w773, "Message"="UI:updateDisplay", "Message Queue"=w774) -> ("error out"=w771:errorcluster)  [unwired: 6 in, 1 out]
      }
      frame "UI:endSubstRef" {
        # "Sets UI state to substitution reference end"
        n280 = call "Enqueue Message.vi"("error in (no error)"=w798, "Message"="UI:endRef", "Message Queue"=w797) -> ("error out"=w796:errorcluster, "dup Message Queue"=w795:refnum<queue>)  [unwired: 7 in]
        n281 = call "Enqueue Message.vi"("error in (no error)"=w796, "Message Data"="Reference completed", "Message"="UI:updateDisplay", "Message Queue"=w795) -> ("error out"=w792:errorcluster)  [unwired: 6 in, 1 out]
      }
      frame "UI:setTab" {
        # "set active page on displayTab."
        n282 = Variant To Data(error in=w807, type=0, Variant=w806) -> (data=w800:i32, error out=w803:errorcluster)
        n283 = control-ref of="Table Key"() -> (w799:refnum<vi>)
        n284 = Unbundle By Name(w804) -> ("Viavi - objectRefs.displayTab"=w801:refnum<vi>)
        n285 = case shown="Default" w800 {
          tunnel: w799 -> [w809 w811]
          frame 1 {
            n286 = property class="Clust (strict)"(reference=w809, "Visible"=TRUE) -> ()  [unwired: 1 in, 2 out]
          }
          frame Default {
            n287 = property class="Clust (strict)"(reference=w811, "Visible"=FALSE) -> ()  [unwired: 1 in, 2 out]
          }
        }
        n288 = property class="TabCtl (strict)"(reference=w801, error in=w803, "Value"=w800) -> (error out=w802:errorcluster)  [unwired: 1 out]
      }
      frame "---------- Device -----------" {
      }
      frame "device:measure" {
        # "Begins a measurement with the selected wavelength.\nQueues a testStatus message to run until measurement is complete.\nRequires wavelength int"
        n289 = Variant To Data(error in=w820, type=0 ("Value"), Variant=w823) -> (data=w825:i32, error out=w814:errorcluster)
        n290 = Unbundle By Name(w815) -> ("Viavi - objectRefs.ResourceNameRef"=w819:refnum<vi>, "Viavi - objectRefs.SlotNumberRef"=w818:refnum<vi>)
        n291 = property class="VISAName"(reference=w819, error in=w814) -> ("Value"=w816:refnum<visa-resource-name>)  [unwired: 2 out]
        n292 = property class="DigNum (strict)"(reference=w818, error in=w814) -> ("Value"=w817:i32)  [unwired: 2 out]
        n293 = call <instrlib>:"Start Measurement.vi"("error in (no error)"=w814, "Wavelength Selection"=w825, "MAP-200 Slot Number"=w817, "VISA resource name"=w816) -> ("error out"=w828:errorcluster)  [unwired: 5 in, 2 out]
        n294 = call "Enqueue Message.vi"("Priority Message? (F)"=TRUE, "error in (no error)"=w828, "Message"="device:testStatus", "Message Queue"=w824) -> ("error out"=w822:errorcluster)  [unwired: 6 in, 1 out]
      }
      frame "device:init" {
        # "Initializes the device to ready for operation"
        n295 = Unbundle By Name(w842) -> ("Viavi - objectRefs.ResourceNameRef"=w844:refnum<vi>, "Viavi - objectRefs.SlotNumberRef"=w843:refnum<vi>)
        n296 = property class="VISAName"(reference=w844, error in=w841) -> ("Value"=w839:refnum<visa-resource-name>)  [unwired: 2 out]
        n297 = property class="DigNum (strict)"(reference=w843, error in=w841) -> ("Value"=w840:i32)  [unwired: 2 out]
        n298 = call <instrlib>:"Configure Function.vi"("error in (no error)"=w841, "Set Function (T = RL Mode)"=TRUE, "MAP-200 Slot Number"=w840, "VISA resource name"=w839) -> ("error out"=w836:errorcluster, "MAP-200 Slot Number out"=w833:i32, "VISA resource name out"=w834:refnum<visa-resource-name>)  [unwired: 5 in]
        n299 = call <instrlib>:"Configure Continuous Mode.vi"("error in (no error)"=w836, "Continuous (On = T)"=FALSE, "MAP-200 Slot Number"=w833, "VISA resource name"=w834) -> ("error out"=w837:errorcluster, "MAP-200 Slot Number out"=w832:i32, "VISA resource name out"=w831:refnum<visa-resource-name>)  [unwired: 5 in]
        n300 = call <instrlib>:"Enable Live Mode.vi"("error in (no error)"=w837, "Enable Live Mode (On = T)"=FALSE, "MAP-200 Slot Number"=w832, "VISA resource name"=w831) -> ("error out"=w838:errorcluster)  [unwired: 5 in, 2 out]
      }
      frame "device:reference" {
        # "Begins a reference with the selected wavelength.\nQueues a testStatus message to run until reference is complete.\nRequires wavelength int"
        n301 = Variant To Data(error in=w857, type=0 ("Value"), Variant=w856) -> (data=w854:i32, error out=w848:errorcluster)
        n302 = Unbundle By Name(w849) -> ("Viavi - objectRefs.ResourceNameRef"=w851:refnum<vi>, "Viavi - objectRefs.SlotNumberRef"=w850:refnum<vi>)
        n303 = property class="VISAName"(reference=w851, error in=w848) -> ("Value"=w847:refnum<visa-resource-name>)  [unwired: 2 out]
        n304 = property class="DigNum (strict)"(reference=w850, error in=w848) -> ("Value"=w846:i32)  [unwired: 2 out]
        n305 = call <instrlib>:"Create Reference.vi"("error in (no error)"=w848, "Wavelength Selection"=w854, "MAP-200 Slot Number"=w846, "VISA resource name"=w847) -> ("error out"=w853:errorcluster)  [unwired: 5 in, 2 out]
        n306 = call "Enqueue Message.vi"("Priority Message? (F)"=TRUE, "error in (no error)"=w853, "Message"="device:testStatus", "Message Queue"=w845) -> ("error out"=w855:errorcluster)  [unwired: 6 in, 1 out]
      }
      frame "device:abort" {
        # "Aborts the last measurement"
        n307 = Unbundle By Name(w864) -> ("Viavi - objectRefs.ResourceNameRef"=w866:refnum<vi>, "Viavi - objectRefs.SlotNumberRef"=w865:refnum<vi>)
        n308 = property class="VISAName"(reference=w866, error in=w861) -> ("Value"=w863:refnum<visa-resource-name>)  [unwired: 2 out]
        n309 = property class="DigNum (strict)"(reference=w865, error in=w861) -> ("Value"=w862:i32)  [unwired: 2 out]
        n310 = call <instrlib>:"Abort Measurement.vi"("error in (no error)"=w861, "MAP-200 Slot Number"=w862, "VISA resource name"=w863) -> ("error out"=w860:errorcluster)  [unwired: 6 in, 2 out]
      }
      frame "device:ILOnly" {
        # "Sets the device to IL Only mode\nDisables device side settings for RL measurement"
        n311 = Variant To Data(error in=w870, type=TRUE, Variant=w869) -> (data=w871:bool, error out=w868:errorcluster)
        n312 = Not(x=w871) -> (.not. x?=w867:bool)
        n313 = Unbundle By Name(w876) -> ("Viavi - objectRefs.ResourceNameRef"=w878:refnum<vi>, "Viavi - objectRefs.SlotNumberRef"=w877:refnum<vi>)
        n314 = property class="VISAName"(reference=w878, error in=w868) -> ("Value"=w874:refnum<visa-resource-name>)  [unwired: 2 out]
        n315 = property class="DigNum (strict)"(reference=w877, error in=w868) -> ("Value"=w875:i32)  [unwired: 2 out]
        n316 = call <instrlib>:"Configure IL Only.vi"("error in (no error)"=w868, "IL Only (On = T)"=w867, "MAP-200 Slot Number"=w875, "VISA resource name"=w874) -> ("error out"=w873:errorcluster)  [unwired: 5 in, 2 out]
      }
      frame "device:multiJumper" {
        # "Sets the device to multi or single jumper mode"
        n317 = Variant To Data(error in=w884, type=TRUE, Variant=w883) -> (data=w885:bool, error out=w880:errorcluster)
        n318 = Unbundle By Name(w887) -> ("Viavi - objectRefs.ResourceNameRef"=w889:refnum<vi>, "Viavi - objectRefs.SlotNumberRef"=w888:refnum<vi>)
        n319 = property class="VISAName"(reference=w889, error in=w880) -> ("Value"=w882:refnum<visa-resource-name>)  [unwired: 2 out]
        n320 = property class="DigNum (strict)"(reference=w888, error in=w880) -> ("Value"=w881:i32)  [unwired: 2 out]
        n321 = call <instrlib>:"Configure MTJ Mode.vi"("error in (no error)"=w880, "Enable Multi Jumper"=w885, "MAP-200 Slot Number"=w881, "VISA resource name"=w882) -> ("error out"=w879:errorcluster)  [unwired: 5 in, 2 out]
      }
      frame "device:takePratio" {
        # "Sets the device to remeasure a new PRatio"
        n322 = call "Enqueue Message.vi"("error in (no error)"=w891, "Message"="UI:startRun", "Message Queue"=w890) -> ("error out"=w892:errorcluster)  [unwired: 7 in, 1 out]
        n323 = Unbundle By Name(w898) -> ("Viavi - objectRefs.ResourceNameRef"=w900:refnum<vi>, "Viavi - objectRefs.SlotNumberRef"=w899:refnum<vi>)
        n324 = property class="VISAName"(reference=w900, error in=w892) -> ("Value"=w896:refnum<visa-resource-name>)  [unwired: 2 out]
        n325 = property class="DigNum (strict)"(reference=w899, error in=w892) -> ("Value"=w897:i32)  [unwired: 2 out]
        n326 = call <instrlib>:"Calibrate Pratio.vi"("error in (no error)"=w892, "MAP-200 Slot Number"=w897, "VISA resource name"=w896) -> ("error out"=w895:errorcluster)  [unwired: 6 in, 2 out]
        n327 = call "Enqueue Message.vi"("Priority Message? (F)"=TRUE, "error in (no error)"=w895, "Message"="device:testStatus", "Message Queue"=w894) -> ("error out"=w901:errorcluster)  [unwired: 6 in, 1 out]
      }
      frame "device:commitPratio" {
        # "Saves the last Pratio measurement if it matches the desired state"
        n328 = call "Enqueue Message.vi"("error in (no error)"=w914, "Message"="UI:endRun", "Message Queue"=w913) -> ("error out"=w907:errorcluster)  [unwired: 7 in, 1 out]
        n329 = Unbundle By Name(w916) -> ("Viavi - objectRefs.ResourceNameRef"=w918:refnum<vi>, "Viavi - objectRefs.SlotNumberRef"=w917:refnum<vi>)
        n330 = property class="VISAName"(reference=w918, error in=w907) -> ("Value"=w909:refnum<visa-resource-name>)  [unwired: 2 out]
        n331 = property class="DigNum (strict)"(reference=w917, error in=w907) -> ("Value"=w908:i32)  [unwired: 2 out]
        n332 = control-ref of="pRatio Array"() -> (w911:refnum<vi>)
        n333 = call <instrlib>:"Commit Pratio.vi"("error in (no error)"=w907, "MAP-200 Slot Number"=w908, "VISA resource name"=w909) -> ("error out"=w906:errorcluster, "MAP-200 Slot Number out"=w905:i32, "VISA resource name out"=w904:refnum<visa-resource-name>)  [unwired: 6 in]
        n334 = call <instrlib>:"Get PRatio.vi"("error in (no error)"=w906, "MAP-200 Slot Number"=w905, "VISA resource name"=w904) -> ("error out"=w910:errorcluster, "Initial Ratio"=w912:dbl[])  [unwired: 4 in, 3 out]
        n335 = property class="Arr (strict)"(reference=w911, "Value"=w912) -> ()  [unwired: 1 in, 2 out]
      }
      frame "device:testStatus" {
        # "Queries the device to determine if it is idle and ready for new input.\nIf not idle, recalls this command after 200ms until in idle status."
        n336 = Unbundle By Name(w920) -> ("Viavi - objectRefs.ResourceNameRef"=w924:refnum<vi>, "Viavi - objectRefs.SlotNumberRef"=w923:refnum<vi>)
        n337 = property class="VISAName"(reference=w924, error in=w919) -> ("Value"=w921:refnum<visa-resource-name>)  [unwired: 2 out]
        n338 = property class="DigNum (strict)"(reference=w923, error in=w919) -> ("Value"=w922:i32)  [unwired: 2 out]
        n339 = call <instrlib>:"Module Status.vi"("error in (no error)"=w919, "MAP-200 Slot Number"=w922, "VISA resource name"=w921) -> ("error out"=w925:errorcluster, "Is Idle (T = Idle)"=w928:bool)  [unwired: 4 in, 3 out]
        n340 = case shown="No Error" w925 {
          selector: w925 -> [w929 w941]
          tunnel: w928 -> [w932 _]
          tunnel: [w931 w941] -> w927
          tunnel: w926 -> [w930 _]
          frame No Error {
            n341 = case shown="False" w932 {
              tunnel: w929 -> [w938 w940]
              tunnel: [w934 w940] -> w931
              tunnel: w930 -> [w936 _]
              frame False {
                n342 = call "Enqueue Message.vi"("Priority Message? (F)"=TRUE, "error in (no error)"=w938, "Message"="device:testStatus", "Message Queue"=w936) -> ("error out"=w935:errorcluster)  [unwired: 6 in, 1 out]
                n343 = call "Stall Data Flow.vim"("value in"=w935, "milliseconds to wait"=200) -> ("value out"=w934:errorcluster)  [unwired: 1 out]
              }
              frame True {
              }
            }
          }
          frame Error {
          }
        }
      }
      frame "device:getMeasData" {
        # "Gets the latest measure data (RL return based on inputs)\nRequires a boolean from selected wavelengths array\nSaves all data to respective arrays, saves last error notifier"
        n344 = Variant To Data(error in=w957, type=TRUE, Variant=w958) -> (data=w953:bool, error out=w952:errorcluster)
        n345 = Unbundle By Name(w956) -> ("Viavi - objectRefs"=w955:T11, "Viavi - objectRefs.TestParamsRef"=w946:refnum<vi>)
        n346 = property class="Clust (strict)"(reference=w946) -> ("Value"=w945:T1)  [unwired: 1 in, 2 out]
        n347 = call "Viavi - Get Measure Data.vi"("error in (no error)"=w952, "Selected Wavelength"=w953, "Warning/Error Params"=w945, "Viavi - strictRefs"=w955) -> ("error out"=w942:errorcluster, "Failure Output"=w944:string, "Output Cluster"=w954:T25)  [unwired: 5 in]
        n348 = Empty String/Path?(string/path=w944) -> (empty?=w943:bool)
        n349 = case shown="False" w943 {
          tunnel: w944 -> [w960 _]
          frame False {
            "Data Error" <- w960
          }
          frame True {
          }
        }
        n350 = Unbundle By Name(w954) -> ("Temp IL Array"=→"Temp IL Array":T2, "Temp RL Array"=→"Temp RL Array":T2, "Temp RL2 Array"=→"Temp RL2 Array":T2, "Temp Power Array"=→"Temp Power Array":T2, "Length Array"=→"Length Array":T2)
      }
      frame "device:getRefData" {
        # "Adds recent or empty data depending on wavelengths used"
        # "Gets the latest reference data of power and length\nRequires a boolean from selected wavelengths array\nSaves all data to Ref Power Array, and only the most recent lengths to Ref Length Array"
        n351 = Unbundle By Name(w973) -> ("Viavi - objectRefs.ResourceNameRef"=w972:refnum<vi>, "Viavi - objectRefs.SlotNumberRef"=w971:refnum<vi>, "Viavi - objectRefs.TestParamsRef"=w963:refnum<vi>, "Viavi - objectRefs.TempRefPowRef"=w970:refnum<vi>, "Viavi - objectRefs.RefLengthRef"=w969:refnum<vi>)
        n352 = Variant To Data(error in=w976, type=TRUE, Variant=w980) -> (data=w979:bool, error out=w961:errorcluster)
        n353 = property class="VISAName"(reference=w972, error in=w961) -> ("Value"=w977:refnum<visa-resource-name>)  [unwired: 2 out]
        n354 = property class="DigNum (strict)"(reference=w971, error in=w961) -> ("Value"=w975:i32)  [unwired: 2 out]
        n355 = property class="Arr (strict)"(reference=w970, error in=w961) -> ("Value"=w974:T2)  [unwired: 2 out]
        n356 = property class="Arr (strict)"(reference=w969, error in=w961) -> ("Value"=w966:T2)  [unwired: 2 out]
        n357 = property class="Clust (strict)"(reference=w963, error in=w961) -> ("Value"=w962:T1)  [unwired: 2 out]
        n358 = case shown="False" w979 {
          tunnel: w977 -> [_ w1006]
          tunnel: [w984 w997] -> w981
          tunnel: w961 -> [w984 w996]
          tunnel: w975 -> [_ w995]
          tunnel: w962 -> [_ w987]
          tunnel: [T21 {"String"="-.--", "Warning"=FALSE, "Fail"=FALSE, "Numeric"=0.0} ("element") w989] -> w965
          tunnel: [T21 {"String"="-.-", "Warning"=FALSE, "Fail"=FALSE, "Numeric"=0.0} ("element") w985] -> w964
          frame False {
          }
          frame True {
            n359 = Unbundle By Name(w987) -> ("Power Param"=w991:T26)
            n360 = call <instrlib>:"Configure Function.vi"("error in (no error)"=w996, "Set Function (T = RL Mode)"=FALSE, "MAP-200 Slot Number"=w995, "VISA resource name"=w1006) -> ("error out"=w999:errorcluster, "MAP-200 Slot Number out"=w1002:i32, "VISA resource name out"=w1005:refnum<visa-resource-name>)  [unwired: 5 in]
            n361 = call <instrlib>:"Get Power.vi"("error in (no error)"=w999, "MAP-200 Slot Number"=w1002, "VISA resource name"=w1005) -> ("error out"=w998:errorcluster, "Power Return (dBm)"=w990:dbl, "MAP-200 Slot Number out"=w1001:i32, "VISA resource name out"=w1004:refnum<visa-resource-name>)  [unwired: 5 in]
            n362 = call "Viavi - Build Cell.vi"("Input Value"=w990, "Parameter Input"=w991) -> ("Single Cell Cluster"=w989:T21)  [unwired: 6 in]
            n363 = Unbundle By Name(w987) -> ("Length Param"=w988:T26)
            n364 = call <instrlib>:"Get DUT Length.vi"("error in (no error)"=w998, "MAP-200 Slot Number"=w1001, "VISA resource name"=w1004) -> ("error out"=w992:errorcluster, "Length Return (m)"=w986:dbl, "MAP-200 Slot Number out"=w1000:i32, "VISA resource name out"=w1003:refnum<visa-resource-name>)  [unwired: 5 in]
            n365 = call "Viavi - Build Cell.vi"("Input Value"=w986, "Parameter Input"=w988) -> ("Single Cell Cluster"=w985:T21)  [unwired: 6 in]
            n366 = call <instrlib>:"Configure Function.vi"("error in (no error)"=w992, "Set Function (T = RL Mode)"=TRUE, "MAP-200 Slot Number"=w1000, "VISA resource name"=w1003) -> ("error out"=w997:errorcluster)  [unwired: 5 in, 2 out]
          }
        }
        n367 = Build Array (concatenate)(w974, w965) -> (→"Temp Ref Power Array":T2)
        n368 = Build Array (concatenate)(w966, w964) -> (→"Ref Length Array":T2)
      }
      frame "device:switch" {
        # "Changes the channel of the connected switch module\nDoes not run if device has no switch\nRequires int defining new channel"
        n369 = Variant To Data(error in=w1012, type=0 ("Switch Channel"), Variant=w1017) -> (data=w1011:i32, error out=w1015:errorcluster)
        n370 = Unbundle By Name(w1010) -> ("Viavi - objectRefs.ResourceNameRef"=w1009:refnum<vi>, "Viavi - objectRefs.SlotNumberRef"=w1008:refnum<vi>, "Viavi - objectRefs.HasSwitchRef"=w1007:refnum<vi>)
        n371 = property class="VISAName"(reference=w1009) -> ("Value"=w1019:refnum<visa-resource-name>)  [unwired: 1 in, 2 out]
        n372 = property class="DigNum (strict)"(reference=w1008) -> ("Value"=w1018:i32)  [unwired: 1 in, 2 out]
        n373 = property class="Bool (strict)"(reference=w1007) -> ("Value"=w1013:bool)  [unwired: 1 in, 2 out]
        n374 = case shown="True" w1013 {
          tunnel: w1019 -> [_ w1025]
          tunnel: w1018 -> [_ w1024]
          tunnel: w1015 -> [w1020 w1023]
          tunnel: [w1020 w1022] -> w1014
          tunnel: w1011 -> [_ w1021]
          frame False {
          }
          frame True {
            n375 = call <instrlib>:"Configure Switch.vi"("error in (no error)"=w1023, "Channel Number"=w1021, "MAP-200 Switch Slot Number"=w1024, "VISA resource name"=w1025) -> ("error out"=w1022:errorcluster)  [unwired: 5 in, 2 out]
          }
        }
      }
    }
  }
  n376 = xnode "Error Ring"() -> ("error out"=w10:errorcluster)
  n377 = while "UI Loop" {
    shift-right: [w1033] -> w9
    shift-left: w10 -> [w1032]
    tunnel: w8 -> [w1031]
    tunnel: "messageQueues" -> [w1029]
    shift-right: [w1026] -> _
    shift-left: w1 -> [w1027]
    stop <- w1034 stop-if-true
    n378 = Unbundle By Name(w1031) -> ("eventRegRef"=w1030:refnum<event-registration>)
    n379 = Unbundle By Name(w1029) -> ("SubVI"=w1028:refnum<queue>)  [unwired: 1 out]
    n380 = event shown="[8] \"Custom RL Cluster\": Mouse Down;  \"Custom RL Cluster\": Value Change" {
      selector: w1030 -> [_ _ _ _ _ _ _ _ _]
      dyn-events: _ -> [_ _ _ _ _ _ _ _ _]
      timeout: _ -> [_ _ _ _ _ _ _ _ _]
      tunnel: [TRUE _ _ _ _ _ _ _ _] -> w1034
      tunnel: [w1036 w1040 _ w1069 w1090 w1105 w1120 w1135 w1150] -> w1033
      tunnel: w1032 -> [w1036 w1039 _ _ w1088 w1103 w1118 w1133 _]
      tunnel: w1028 -> [_ w1038 _ _ w1091 w1106 w1121 w1136 w1149]
      tunnel: w1027 -> [w1035 w1045 w1056 w1081 w1096 w1111 w1126 w1141 w1154]
      tunnel: [w1035 w1045 w1056 w1081 w1096 w1111 w1126 w1141 w1154] -> w1026
      event User Event {
        # "Sends the event to stop the event handler while loop"
        n381 = event-data() -> ()  [unwired: 1 in, 1 out]
      }
      event "Measure pRatio": Value Change {
        # "Forces a new pRatio measurement"
        n382 = event-data() -> ()  [unwired: 1 in, 1 out]
        n383 = call "Enqueue Message.vi"("error in (no error)"=w1039, "Message"="device:takePratio", "Message Queue"=w1038) -> ("error out"=w1044:errorcluster, "dup Message Queue"=w1043:refnum<queue>)  [unwired: 7 in]
        n384 = call "Enqueue Message.vi"("error in (no error)"=w1044, "Message"="device:commitPratio", "Message Queue"=w1043) -> ("error out"=w1040:errorcluster)  [unwired: 7 in, 1 out]
      }
      event "RL2 Standard": Value Change {
        # "Sets the standard used for the RL2 measurements"
        n385 = event-data() -> ()  [unwired: 1 in, 1 out]
        n386 = Unbundle By Name(w1056) -> ("Viavi - objectRefs.TestParamsRef"=w1047:refnum<vi>, "Viavi - objectRefs.RL2StandardRef"=w1050:refnum<vi>)
        n387 = call "IL-RL Standards.vi"("Input New Standard"=T20 {"Standard Name"="", "Max IL to Pass (dB)"=0.0, "Min RL to Pass (dB)"=0.0}) -> ("IL RL Standards"=w1052:T27)  [unwired: 8 in, 1 out]
        n388 = case shown="1, 4" "RL2 Standard" {
          selector: "RL2 Standard" -> [_ _ _ _ w1066]
          tunnel: w1052 -> [_ _ _ _ w1068]
          tunnel: [T20 {"Standard Name"="No Standard Set", "Max IL to Pass (dB)"=inf, "Min RL to Pass (dB)"=-inf} ("IL RL Standards") T20 {"Standard Name"="No Standard Set", "Max IL to Pass (dB)"=inf, "Min RL to Pass (dB)"=-inf} ("IL RL Standards") T20 {"Standard Name"="No Standard Set", "Max IL to Pass (dB)"=inf, "Min RL to Pass (dB)"=-inf} ("IL RL Standards") w1063 w1067] -> w1049
          tunnel: w1050 -> [_ w1058 _ _ _]
          frame 0 {
          }
          frame 1, 4 {
            n389 = property class="Ring (strict)"(reference=w1058, "Value"=u16 0) -> ()  [unwired: 1 in, 2 out]
          }
          frame 2 {
          }
          frame 3 {
            n390 = call "Custom Standard.vi"("IL Enable"=FALSE) -> ("Output Custom"=w1063:T20)  [unwired: 7 in]
          }
          frame Default {
            n391 = Subtract(x=w1066, y=u16 5) -> (x-y=w1064:u16)
            n392 = Index Array(array=w1068, index=w1064) -> (element=w1067:T20)
          }
        }
        n393 = property class="Clust (strict)"(reference=w1047) -> (reference out=w1054:refnum<vi>, "Value"=w1055:T1)  [unwired: 1 in, 1 out]
        n394 = Unbundle By Name(w1049) -> ("Min RL to Pass (dB)"=w1048:dbl)
        n395 = Bundle By Name(cluster=w1055, "RL2 Param.Fail Low"=w1048) -> (w1053:T1)
        n396 = property class="Clust (strict)"(reference=w1054, "Value"=w1053) -> ()  [unwired: 1 in, 2 out]
      }
      event "IL Warnings Enable", "IL Warning Values": Value Change {
        n397 = event-data() -> ()  [unwired: 1 in, 1 out]
        n398 = Unbundle By Name(w1081) -> ("Viavi - objectRefs.TestParamsRef"=w1080:refnum<vi>)
        n399 = case shown="True" "IL Warnings Enable" {
          tunnel: [inf ("IL Max") w1085] -> w1076
          tunnel: [0.0 ("IL Min") w1084] -> w1075
          frame False {
          }
          frame True {
            n400 = Unbundle By Name("IL Warning Values") -> ("IL Min"=w1084:dbl, "IL Max"=w1085:dbl)
          }
        }
        n401 = property class="Clust (strict)"(reference=w1080) -> (reference out=w1077:refnum<vi>, "Value"=w1079:T1)  [unwired: 1 in, 1 out]
        n402 = Bundle By Name(cluster=w1079, "IL Param.Fail Low"=w1075, "IL Param.Fail High"=w1076) -> (w1078:T1)
        n403 = Select(t=0, s="IL Warnings Enable", f=2) -> (s? t:f=w1071:i32)
        n404 = control-ref of="IL Warning Values"() -> (w1070:refnum<vi>)
        n405 = property class="Clust (strict)"(reference=w1070, "DisabledEnum"=w1071) -> (error out=w1069:errorcluster)  [unwired: 1 in, 1 out]
        n406 = property class="Clust (strict)"(reference=w1077, "Value"=w1078) -> ()  [unwired: 1 in, 2 out]
      }
      event "Input Image": Mouse Down {
        # "Changes the RL Preset value when image is clicked"
        n407 = event-data() -> ()  [unwired: 1 in, 1 out]
        n408 = Unbundle By Name(w1096) -> ("Viavi - objectRefs.RLPresetRef"=w1095:refnum<vi>)
        n409 = property class="RadioBtnsControl (strict)"(reference=w1095, error in=w1088) -> (error out=w1089:errorcluster, "DisabledEnum"=w1094:T14)  [unwired: 1 out]
        n410 = Equal To 0?(x=w1094) -> (x = 0?=w1093:bool)
        n411 = case shown="True" w1093 {
          tunnel: w1095 -> [_ w1100]
          tunnel: [w1097 w1099] -> w1087
          tunnel: w1089 -> [w1097 w1098]
          frame False {
          }
          frame True {
            n412 = property class="RadioBtnsControl (strict)"(reference=w1100, error in=w1098, "Value"=T5."Left Anchor") -> (error out=w1099:errorcluster)  [unwired: 1 out]
          }
        }
        n413 = call "Enqueue Message.vi"("error in (no error)"=w1087, "Message"="macro:preset", "Message Queue"=w1091) -> ("error out"=w1090:errorcluster)  [unwired: 7 in, 1 out]
      }
      event "Output Image": Mouse Down {
        # "Changes the RL Preset value when image is clicked"
        n414 = event-data() -> ()  [unwired: 1 in, 1 out]
        n415 = Unbundle By Name(w1111) -> ("Viavi - objectRefs.RLPresetRef"=w1110:refnum<vi>)
        n416 = property class="RadioBtnsControl (strict)"(reference=w1110, error in=w1103) -> (error out=w1104:errorcluster, "DisabledEnum"=w1109:T14)  [unwired: 1 out]
        n417 = Equal To 0?(x=w1109) -> (x = 0?=w1108:bool)
        n418 = case shown="True" w1108 {
          tunnel: w1110 -> [_ w1115]
          tunnel: [w1112 w1114] -> w1102
          tunnel: w1104 -> [w1112 w1113]
          frame False {
          }
          frame True {
            n419 = property class="RadioBtnsControl (strict)"(reference=w1115, error in=w1113, "Value"=T5."Right Anchor") -> (error out=w1114:errorcluster)  [unwired: 1 out]
          }
        }
        n420 = call "Enqueue Message.vi"("error in (no error)"=w1102, "Message"="macro:preset", "Message Queue"=w1106) -> ("error out"=w1105:errorcluster)  [unwired: 7 in, 1 out]
      }
      event "Between Image": Mouse Down {
        # "Changes the RL Preset value when image is clicked"
        n421 = event-data() -> ()  [unwired: 1 in, 1 out]
        n422 = Unbundle By Name(w1126) -> ("Viavi - objectRefs.RLPresetRef"=w1125:refnum<vi>)
        n423 = property class="RadioBtnsControl (strict)"(reference=w1125, error in=w1118) -> (error out=w1119:errorcluster, "DisabledEnum"=w1124:T14)  [unwired: 1 out]
        n424 = Equal To 0?(x=w1124) -> (x = 0?=w1123:bool)
        n425 = case shown="True" w1123 {
          tunnel: w1125 -> [_ w1130]
          tunnel: [w1127 w1129] -> w1117
          tunnel: w1119 -> [w1127 w1128]
          frame False {
          }
          frame True {
            n426 = property class="RadioBtnsControl (strict)"(reference=w1130, error in=w1128, "Value"=T5."Center Anchor") -> (error out=w1129:errorcluster)  [unwired: 1 out]
          }
        }
        n427 = call "Enqueue Message.vi"("error in (no error)"=w1117, "Message"="macro:preset", "Message Queue"=w1121) -> ("error out"=w1120:errorcluster)  [unwired: 7 in, 1 out]
      }
      event "Both Image": Mouse Down {
        # "Changes the RL Preset value when image is clicked"
        n428 = event-data() -> ()  [unwired: 1 in, 1 out]
        n429 = Unbundle By Name(w1141) -> ("Viavi - objectRefs.RLPresetRef"=w1140:refnum<vi>)
        n430 = property class="RadioBtnsControl (strict)"(reference=w1140, error in=w1133) -> (error out=w1134:errorcluster, "DisabledEnum"=w1139:T14)  [unwired: 1 out]
        n431 = Equal To 0?(x=w1139) -> (x = 0?=w1138:bool)
        n432 = case shown="True" w1138 {
          tunnel: w1140 -> [_ w1145]
          tunnel: [w1142 w1144] -> w1132
          tunnel: w1134 -> [w1142 w1143]
          frame False {
          }
          frame True {
            n433 = property class="RadioBtnsControl (strict)"(reference=w1145, error in=w1143, "Value"=T5."Left/Right Anchor") -> (error out=w1144:errorcluster)  [unwired: 1 out]
          }
        }
        n434 = call "Enqueue Message.vi"("error in (no error)"=w1132, "Message"="macro:preset", "Message Queue"=w1136) -> ("error out"=w1135:errorcluster)  [unwired: 7 in, 1 out]
      }
      event "Custom RL Cluster": Mouse Down; "Custom RL Cluster": Value Change {
        # "Sets the custom RL Preset settings based on the last used setting"
        n435 = event-data() -> ()  [unwired: 1 in, 1 out]
        n436 = Unbundle By Name(w1154) -> ("Viavi - objectRefs.RLPresetRef"=w1153:refnum<vi>)
        n437 = property class="RadioBtnsControl (strict)"(reference=w1153) -> (reference out=w1151:refnum<vi>, "Value"=w1152:T5, "DisabledEnum"=w1148:T14)  [unwired: 1 in, 1 out]
        n438 = Equal To 0?(x=w1148) -> (x = 0?=w1147:bool)
        n439 = case shown="True" w1147 {
          tunnel: w1152 -> [_ w1171]
          tunnel: w1151 -> [_ w1155]
          tunnel: [_ w1163] -> w1150
          tunnel: w1149 -> [_ w1161]
          frame False {
          }
          frame True {
            n440 = control-ref of="Int Mode"() -> (w1170:refnum<vi>)
            n441 = control-ref of="RL 1 A"() -> (w1169:refnum<vi>)
            n442 = control-ref of="RL 1 B"() -> (w1168:refnum<vi>)
            n443 = control-ref of="RL 2 A"() -> (w1167:refnum<vi>)
            n444 = control-ref of="RL 2 B"() -> (w1166:refnum<vi>)
            n445 = case shown="\"Center Anchor\"" w1171 {
              tunnel: w1170 -> [w1181 w1193 w1205 w1217 _]
              tunnel: w1169 -> [w1180 w1192 w1204 w1216 _]
              tunnel: w1168 -> [w1179 w1191 w1203 w1215 _]
              tunnel: w1167 -> [w1178 w1190 w1202 w1214 _]
              tunnel: w1166 -> [w1177 w1189 w1201 w1213 _]
              tunnel: [FALSE FALSE FALSE TRUE w1219] -> w1159
              tunnel: [1 2 3 4 w1220] -> w1158
              frame "Left Anchor" {
                w1175 = 0.0
                w1182 = 2
                n446 = property class="Bool (strict)"(reference=w1181, "Value"=FALSE) -> ()  [unwired: 1 in, 2 out]
                n447 = property class="DigNum (strict)"(reference=w1180, "Value"=-0.25) -> ()  [unwired: 1 in, 2 out]
                n448 = property class="DigNum (strict)"(reference=w1179, "Value"=0.25) -> ()  [unwired: 1 in, 2 out]
                n449 = property class="DigNum (strict)"(reference=w1178, "Value"=w1175, "DisabledEnum"=w1182) -> ()  [unwired: 1 in, 2 out]
                n450 = property class="DigNum (strict)"(reference=w1177, "Value"=w1175, "DisabledEnum"=w1182) -> ()  [unwired: 1 in, 2 out]
              }
              frame "Right Anchor" {
                w1187 = 0.0
                w1194 = 2
                n451 = property class="Bool (strict)"(reference=w1193, "Value"=FALSE) -> ()  [unwired: 1 in, 2 out]
                n452 = property class="DigNum (strict)"(reference=w1192, "Value"=-0.25) -> ()  [unwired: 1 in, 2 out]
                n453 = property class="DigNum (strict)"(reference=w1191, "Value"=0.25) -> ()  [unwired: 1 in, 2 out]
                n454 = property class="DigNum (strict)"(reference=w1190, "Value"=w1187, "DisabledEnum"=w1194) -> ()  [unwired: 1 in, 2 out]
                n455 = property class="DigNum (strict)"(reference=w1189, "Value"=w1187, "DisabledEnum"=w1194) -> ()  [unwired: 1 in, 2 out]
              }
              frame "Center Anchor" {
                w1199 = 0.0
                w1206 = 2
                n456 = property class="Bool (strict)"(reference=w1205, "Value"=TRUE) -> ()  [unwired: 1 in, 2 out]
                n457 = property class="DigNum (strict)"(reference=w1204, "Value"=0.5) -> ()  [unwired: 1 in, 2 out]
                n458 = property class="DigNum (strict)"(reference=w1203, "Value"=-0.5) -> ()  [unwired: 1 in, 2 out]
                n459 = property class="DigNum (strict)"(reference=w1202, "Value"=w1199, "DisabledEnum"=w1206) -> ()  [unwired: 1 in, 2 out]
                n460 = property class="DigNum (strict)"(reference=w1201, "Value"=w1199, "DisabledEnum"=w1206) -> ()  [unwired: 1 in, 2 out]
              }
              frame "Left/Right Anchor" {
                w1209 = 0.25
                w1218 = 0
                w1208 = -0.25
                n461 = property class="Bool (strict)"(reference=w1217, "Value"=FALSE) -> ()  [unwired: 1 in, 2 out]
                n462 = property class="DigNum (strict)"(reference=w1216, "Value"=w1208) -> ()  [unwired: 1 in, 2 out]
                n463 = property class="DigNum (strict)"(reference=w1215, "Value"=w1209) -> ()  [unwired: 1 in, 2 out]
                n464 = property class="DigNum (strict)"(reference=w1214, "Value"=w1208, "DisabledEnum"=w1218) -> ()  [unwired: 1 in, 2 out]
                n465 = property class="DigNum (strict)"(reference=w1213, "Value"=w1209, "DisabledEnum"=w1218) -> ()  [unwired: 1 in, 2 out]
              }
              frame Default {
                n466 = control-ref of="Custom RL Cluster"() -> (w1222:refnum<vi>)
                n467 = property class="Clust (strict)"(reference=w1222) -> ("Value"=w1221:T4)  [unwired: 1 in, 2 out]
                n468 = Unbundle By Name(w1221) -> ("RL Method"=w1220:u16, "Enable RL2"=w1219:bool)
              }
            }
            n469 = control-ref of="RL Method"() -> (w1156:refnum<vi>)
            n470 = control-ref of="Enable RL2"() -> (w1160:refnum<vi>)
            n471 = property class="RadioBtnsControl (strict)"(reference=w1155, "Value"=T5."Custom") -> (error out=w1162:errorcluster)  [unwired: 1 in, 1 out]
            n472 = property class="Ring (strict)"(reference=w1156, "Value"=w1158, "Visible"=TRUE) -> ()  [unwired: 1 in, 2 out]
            n473 = property class="Bool (strict)"(reference=w1160, "Value"=w1159) -> ()  [unwired: 1 in, 2 out]
            n474 = call "Enqueue Message.vi"("error in (no error)"=w1162, "Message"="macro:preset", "Message Queue"=w1161) -> ("error out"=w1163:errorcluster)  [unwired: 7 in, 1 out]
          }
        }
      }
    }
  }
  n475 = call "Destroy User Event - Stop.vi"("error in (no error)"=w13, "userEvents"=w8) -> ("error out"=w12:errorcluster)  [unwired: 9 in]
  n476 = Merge Errors(w9, w12) -> (→"error out":errorcluster)
